vi "日志信息出发送队列 (子VI).vi"(11 "queue out":refnum<queue>) -> (0 "错误输出":errorcluster)   [LabVIEW 2016, in "数据传输系统.lvlib"]
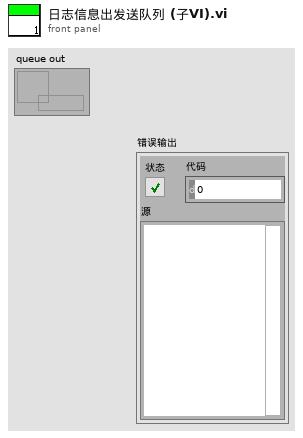
[diagram p1: front panel]
types:
  T1 = enum16{"空白测试", "跨度核查", "标样核查", "加标回收", "平行样", "集成干预"}
  T2 = typedef "数据传输系统.lvlib/应用环境.ctl" = enum16{"STD", "GB212", "婉仪平台"}
  T3 = cluster{"氨氮零点核查索引起始时间":string, "总磷零点核查索引起始时间":string, "总氮零点核查索引起始时间":string, "CODMn零点核查索引起始时间":string, "CODCr零点核查索引起始时间":string, "亚硝酸盐零点核查索引起始时间":string, "硫化物零点核查索引起始时间":string, "ORP零点核查索引起始时间":string, "氟化物零点核查索引起始时间":string, "挥发酚零点核查索引起始时间":string}
  T4 = cluster{"数组[0]":string, "数组[1]":string, "数组[2]":string, "数组[3]":string, "数组[4]":string, "数组[5]":string, "数组[6]":string, "数组[7]":string, "数组[8]":string, "数组[9]":string}
  T5 = cluster{"PH":string[][], "CODCr":string[][], "氨氮":string[][], "CODMn":string[][], "总氮":string[][], "总磷":string[][], "电导率":string[][], "水温":string[][], "DO":string[][], "浊度":string[][], "叶绿素":string[][], "藻密度":string[][], "铜":string[][], "盐度":string[][], "水位":string[][], "流速":string[][], "瞬时流量":string[][], "累积流量":string[][], "亚硝酸盐":string[][], "硫化物":string[][], "ORP":string[][], "铅":string[][], "镉":string[][], "锌":string[][], "镍":string[][], "锰":string[][], "汞":string[][], "气温":string[][], "气压":string[][], "风速":string[][], "风向":string[][], "盐度 2":string[][], "磷酸盐":string[][], "硝氮":string[][], "氟化物":string[][], "挥发酚":string[][], "氯化物":string[][], "蓝绿藻":string[][]}
  T6 = cluster{"氨氮跨度核查索引起始时间":string, "总磷跨度核查索引起始时间":string, "总氮跨度核查索引起始时间":string, "CODMn跨度核查索引起始时间":string, "CODCr跨度核查索引起始时间":string, "亚硝酸盐跨度核查索引起始时间":string, "硫化物跨度核查索引起始时间":string, "ORP跨度核查索引起始时间":string, "氟化物跨度核查索引起始时间":string, "挥发酚跨度核查索引起始时间":string}
  T7 = cluster{"氨氮标样核查索引起始时间":string, "总磷标样核查索引起始时间":string, "总氮标样核查索引起始时间":string, "CODMn标样核查索引起始时间":string, "CODCr标样核查索引起始时间":string, "DO标样核查索引起始时间":string, "PH标样核查索引起始时间":string, "比电导率标样核查索引起始时间":string, "水温标样核查索引起始时间":string, "浊度标样核查索引起始时间":string, "叶绿素a标样核查索引起始时间":string, "藻密度标样核查索引起始时间":string, "亚硝酸盐标样核查索引起始时间":string, "硫化物标样核查索引起始时间":string, "ORP标样核查索引起始时间":string, "氟化物标样核查索引起始时间":string, "挥发酚标样核查索引起始时间":string, "氯化物标样核查索引起始时间":string}
  T8 = cluster{"数组[0]":string, "数组[1]":string, "数组[2]":string, "数组[3]":string, "数组[4]":string, "数组[5]":string, "数组[6]":string, "数组[7]":string, "数组[8]":string, "数组[9]":string, "数组[10]":string, "数组[11]":string, "数组[12]":string, "数组[13]":string, "数组[14]":string, "数组[15]":string, "数组[16]":string, "数组[17]":string}
  T9 = cluster{"氨氮加标回收索引起始时间":string, "总磷加标回收索引起始时间":string, "总氮加标回收索引起始时间":string, "CODMn加标回收索引起始时间":string, "CODCr加标回收索引起始时间":string, "氟化物加标回收索引起始时间":string, "挥发酚加标回收索引起始时间":string}
  T10 = cluster{"[0]":string, "[1]":string, "[2]":string, "[3]":string, "[4]":string, "[5]":string, "[6]":string}
  T11 = cluster{"氨氮平行样索引起始时间":string, "总磷平行样索引起始时间":string, "总氮平行样索引起始时间":string, "CODMn平行样索引起始时间":string, "CODCr平行样索引起始时间":string, "氟化物平行样索引起始时间":string, "挥发酚平行样索引起始时间":string}
  T12 = cluster{"氨氮集成干预索引起始时间":string, "总磷集成干预索引起始时间":string, "总氮集成干预索引起始时间":string, "CODMn集成干预索引起始时间":string, "CODCr集成干预索引起始时间":string, "DO集成干预索引起始时间":string, "PH集成干预索引起始时间":string, "比电导率集成干预索引起始时间":string, "水温集成干预索引起始时间":string, "浊度集成干预索引起始时间":string, "叶绿素a集成干预索引起始时间":string, "藻密度集成干预索引起始时间":string, "亚硝酸盐集成干预索引起始时间":string, "硫化物集成干预索引起始时间":string, "ORP集成干预索引起始时间":string, "氟化物集成干预索引起始时间":string, "挥发酚集成干预索引起始时间":string, "氯化物集成干预索引起始时间":string}
  T13 = cluster{"[0]":string, "[1]":string, "[2]":string, "[3]":string, "[4]":string, "[5]":string, "[6]":string, "[7]":string, "[8]":string, "[9]":string, "[10]":string, "[11]":string, "[12]":string, "[13]":string, "[14]":string, "[15]":string, "[16]":string, "[17]":string}
  T14 = cluster{"氨氮仪器日志索引起始时间":string, "总磷仪器日志索引起始时间":string, "总氮仪器日志索引起始时间":string, "CODMn仪器日志索引起始时间":string, "CODCr仪器日志索引起始时间":string, "系统仪器日志索引起始时间":string, "氟化物仪器日志索引起始时间":string, "挥发酚仪器日志索引起始时间":string}
  T15 = cluster{"[0]":string, "[1]":string, "[2]":string, "[3]":string, "[4]":string, "[5]":string, "[6]":string, "[7]":string}
  T16 = cluster{"氨氮报警信息索引起始时间":string, "总磷报警信息索引起始时间":string, "总氮报警信息索引起始时间":string, "CODMn报警信息索引起始时间":string, "CODCr报警信息索引起始时间":string, "DO报警信息索引起始时间":string, "PH报警信息索引起始时间":string, "比电导率报警信息索引起始时间":string, "水温报警信息索引起始时间":string, "浊度报警信息索引起始时间":string, "叶绿素报警信息索引起始时间":string, "系统报警信息索引起始时间":string, "氟化物报警信息索引起始时间":string, "挥发酚报警信息索引起始时间":string}
  T17 = cluster{"[0]":string, "[1]":string, "[2]":string, "[3]":string, "[4]":string, "[5]":string, "[6]":string, "[7]":string, "[8]":string, "[9]":string, "[10]":string, "[11]":string, "[12]":string, "[13]":string}
  T18 = cluster{"氨氮仪器参数索引起始时间":string, "总磷仪器参数索引起始时间":string, "总氮仪器参数索引起始时间":string, "CODMn仪器参数索引起始时间":string, "CODCr仪器参数索引起始时间":string, "DO仪器参数索引起始时间":string, "PH仪器参数索引起始时间":string, "比电导率仪器参数索引起始时间":string, "水温仪器参数索引起始时间":string, "浊度仪器参数索引起始时间":string, "叶绿素a仪器参数索引起始时间":string, "藻密度仪器参数索引起始时间":string, "ORP仪器参数索引起始时间":string, "氟化物仪器参数索引起始时间":string, "挥发酚仪器参数索引起始时间":string}
  T19 = cluster{"[0]":string, "[1]":string, "[2]":string, "[3]":string, "[4]":string, "[5]":string, "[6]":string, "[7]":string, "[8]":string, "[9]":string, "[10]":string, "[11]":string, "[12]":string, "[13]":string, "[14]":string}
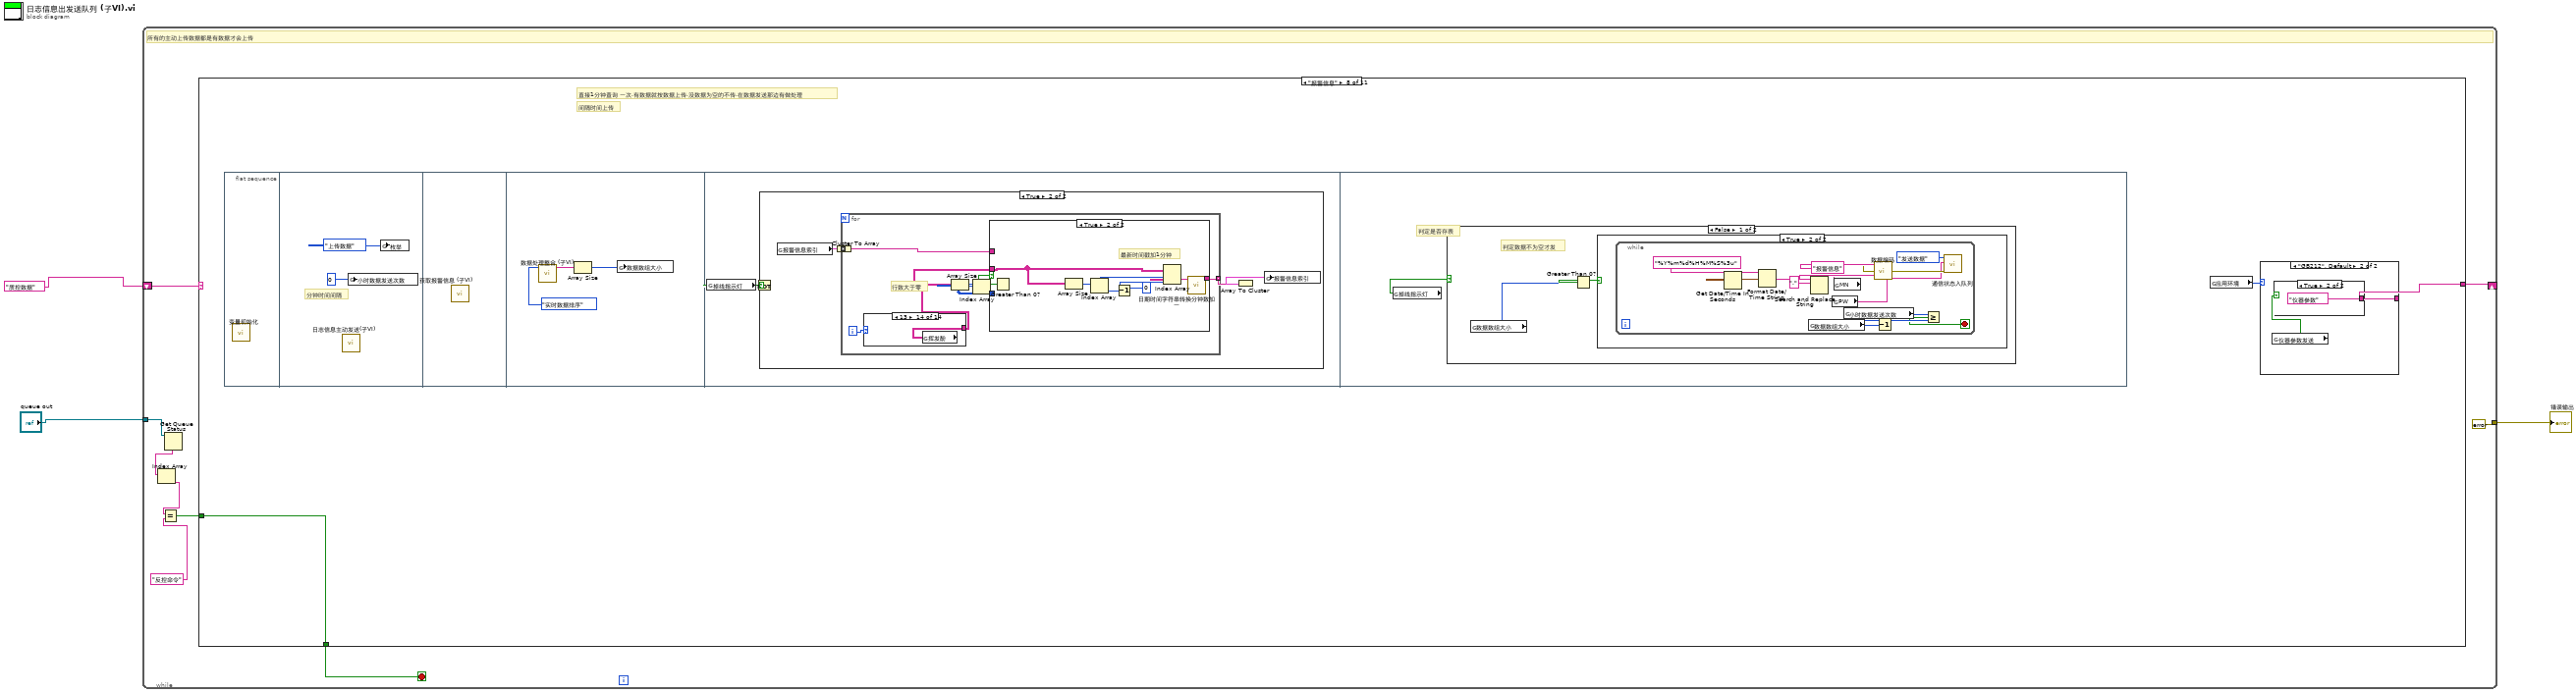
[diagram p0: block diagram]
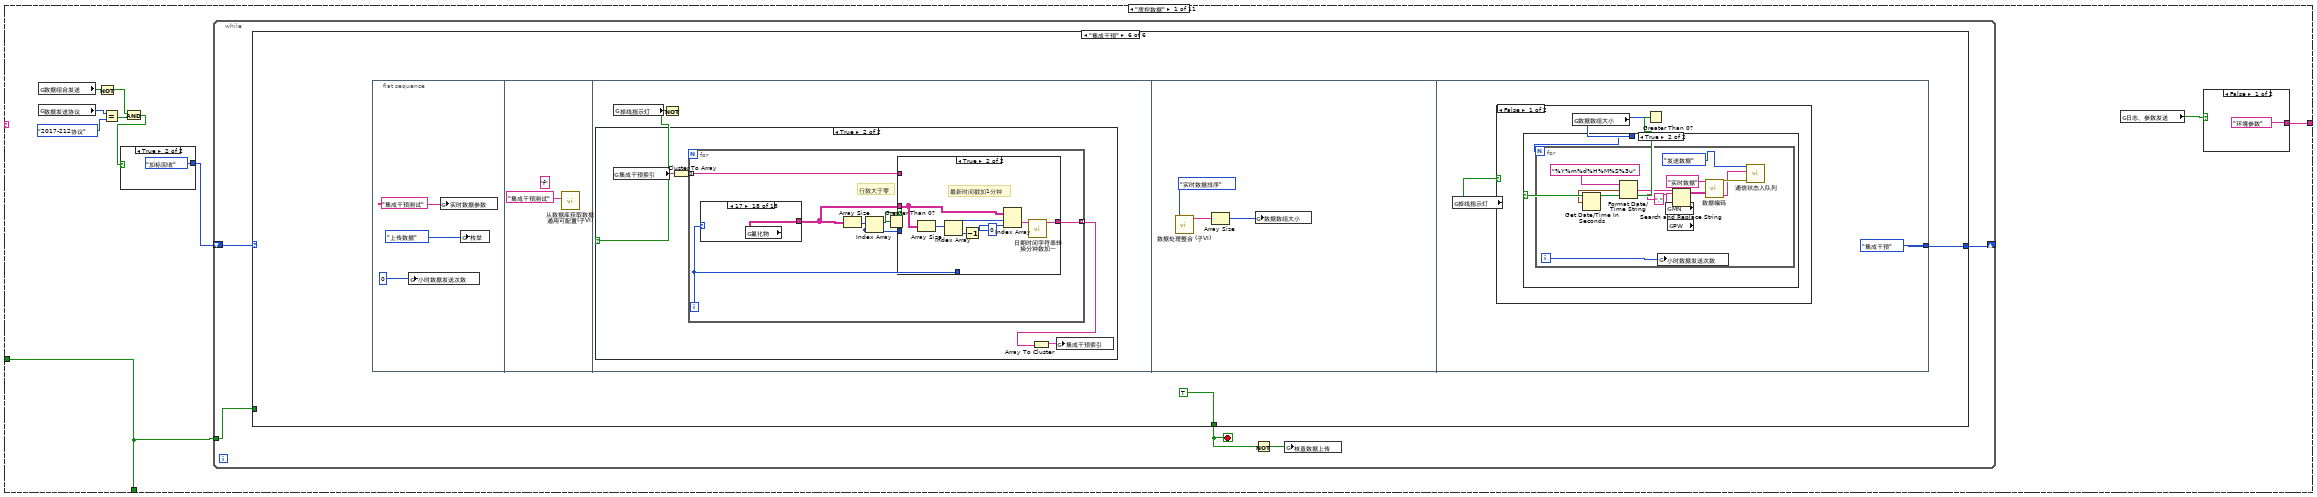
[diagram p2: hidden frame]
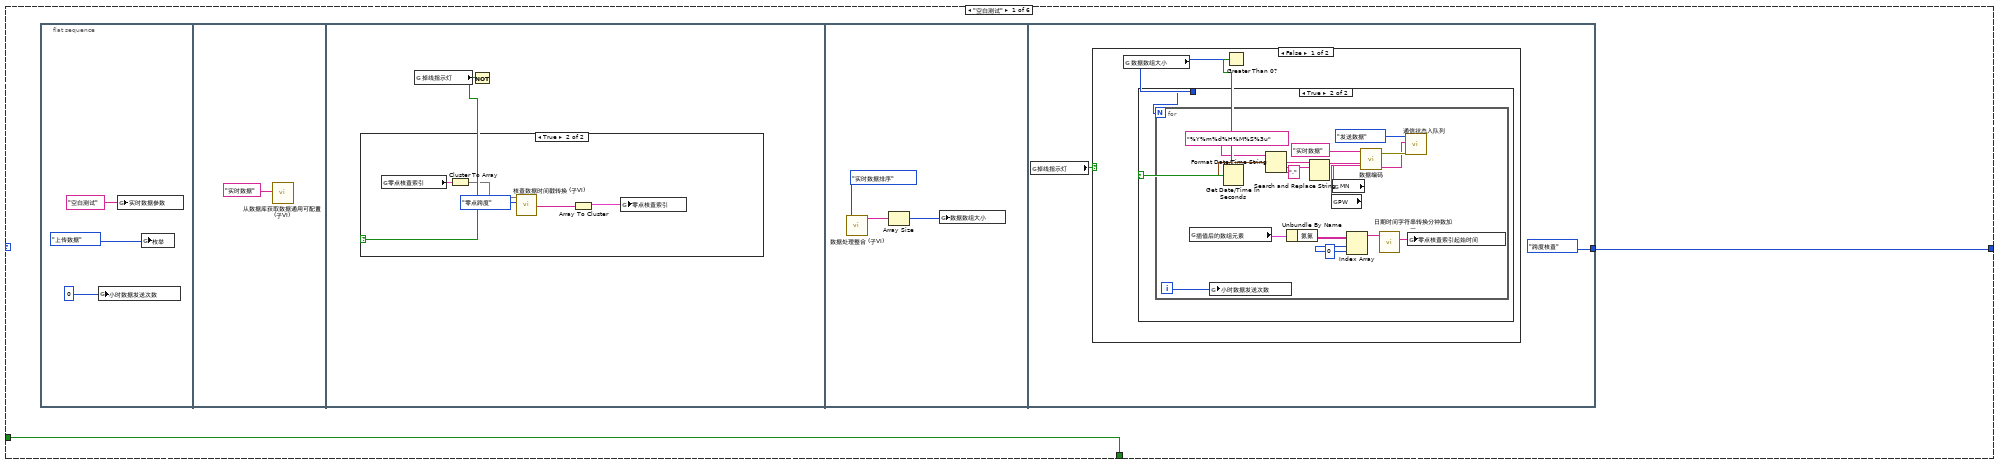
[diagram p3: hidden frame]
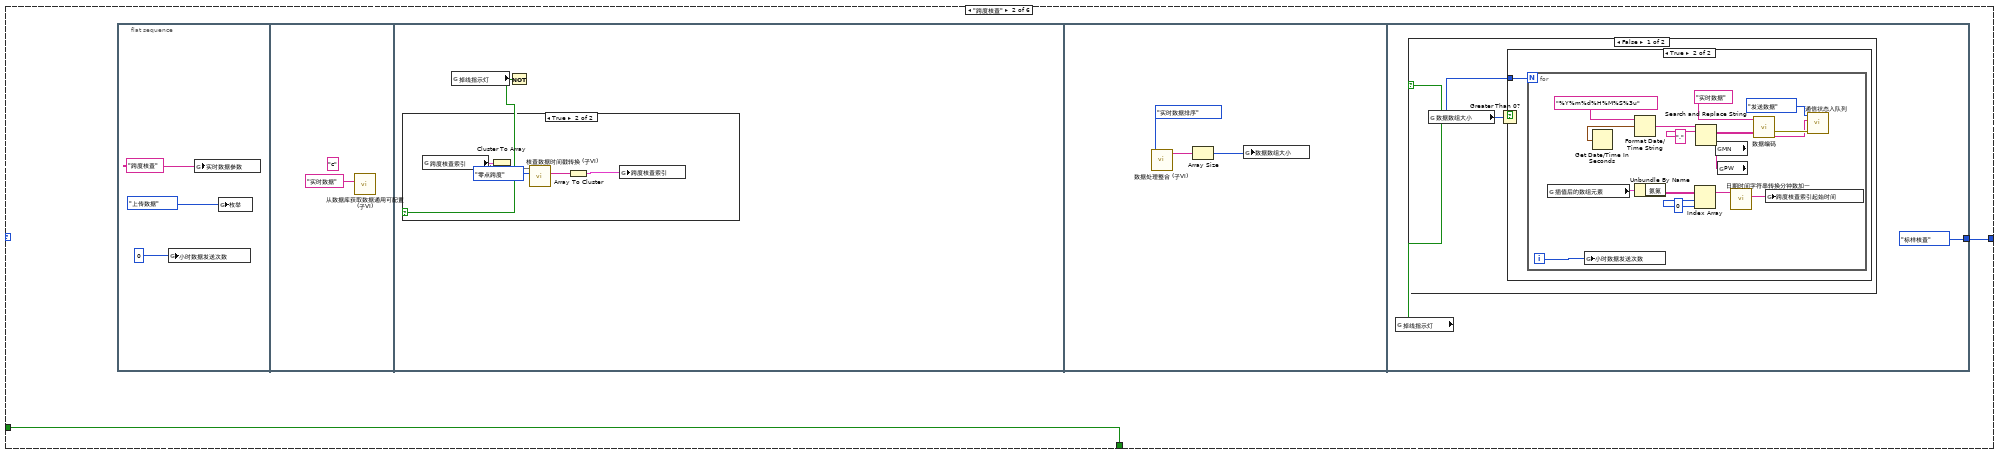
[diagram p7: hidden frame]
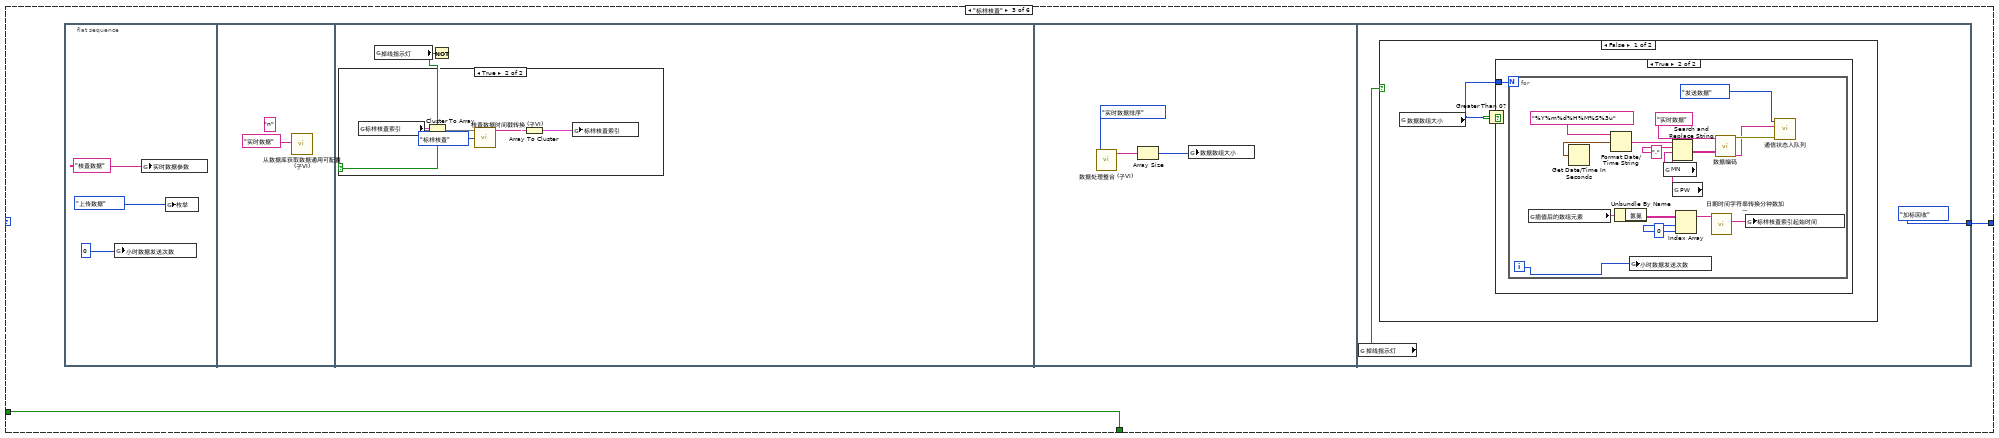
[diagram p11: hidden frame]
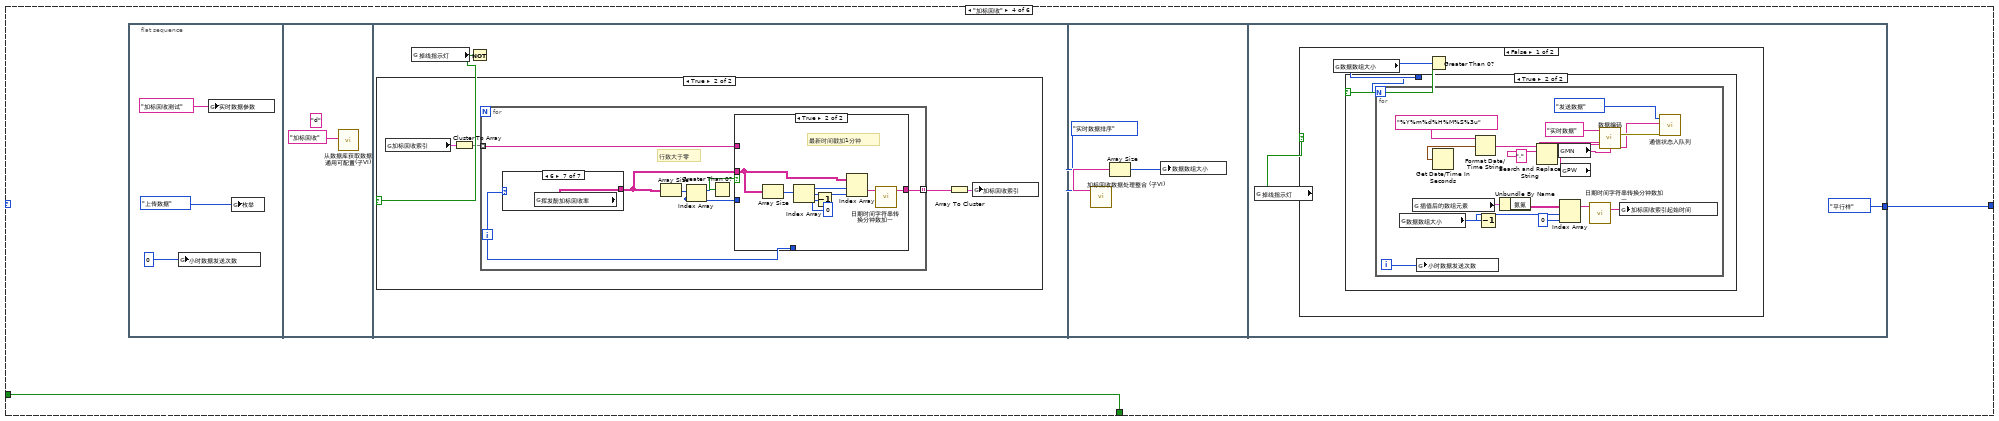
[diagram p15: hidden frame]
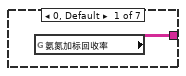
[diagram p17: hidden frame]
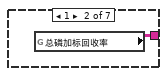
[diagram p18: hidden frame]
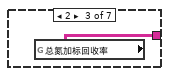
[diagram p19: hidden frame]
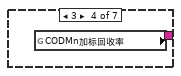
[diagram p20: hidden frame]
diagram:
  n1 = while "While循环" {
    shift-right: [w11] -> _
    shift-left: "质控数据" ("组合框") -> [w12]
    tunnel: [errorcluster {"status"=FALSE, "code"=0, "source"=""} ("错误输出")] -> w3
    tunnel: "queue out" -> [w8]
    stop <- w9 stop-if-true
    # "所有的主动上传数据都是有数据才会上传"
    n2 = Get Queue Status(queue=w8) -> (elements=w7:string[])  [unwired: 2 in, 7 out]
    n3 = Index Array(array=w7) -> (element=w6:string)  [unwired: 1 in]
    n4 = Equal?(x=w6, y="反控命令" ("元素")) -> (x = y?=w4:bool)
    n5 = case shown="\"报警信息\"" w12 {
      tunnel: [w22 w327 "系统状态" ("组合框") w430 "测量周期" ("组合框") "超标留样" ("组合框") "报警信息" ("组合框") w575 w642 "环境参数" ("组合框") "环境参数" ("组合框")] -> w11
      tunnel: [w13 w326 w384 w428 w454 w488 w553 w574 w641 w688 TRUE] -> w9
      tunnel: w4 -> [w13 w326 w384 w428 w454 w488 w553 w574 w641 w688 _]
      frame "质控数据" {
        n6 = global read "断电保存全局.vi" "数据组合发送"() -> (w17:bool)
        n7 = global read "断电保存全局.vi" "数据发送协议"() -> (w20:enum16{"2005-212协议", "2017-212协议"})
        n8 = Not(x=w17) -> (.not. x?=w16:bool)
        n9 = Equal?(x=w20, y=enum16{"2005-212协议", "2017-212协议"}."2017-212协议" ("数据发送协议")) -> (x = y?=w18:bool)
        n10 = And(x=w16, y=w18) -> (x .and. y?=w15:bool)
        n11 = case shown="True" w15 {
          tunnel: [T1."空白测试" T1."加标回收"] -> w14
          frame False {
          }
          frame True {
          }
        }
        n12 = while {
          shift-right: [w26] -> _
          shift-left: w14 -> [w27]
          tunnel: w13 -> [w23]
          stop <- w24 stop-if-true
          n13 = case shown="\"集成干预\"" w27 {
            tunnel: [w28 w66 w104 w142 w203 TRUE] -> w24
            tunnel: [w29 w67 w105 w143 w204 w257] -> w26
            tunnel: w23 -> [w28 w66 w104 w142 w203 _]
            frame "空白测试" {
              n14 = flat-sequence {
                tunnel: [T1."跨度核查"] -> w29
                frame #0 {
                  n15 = global write "全局 小时数据发送次数.vi" "小时数据发送次数"(0 ("小时数据发送次数")) -> ()
                  n16 = global write "全局 实时数据参数.vi" "实时数据参数"("空白测试") -> ()
                  n17 = global write "全局1.vi" "枚举"(enum16{"返回请求应答", "上传数据", "返回执行结果"}."上传数据" ("枚举")) -> ()
                }
                frame #1 {
                  n18 = call "从数据库获取数据通用可配置(子VI).vi"("table输入"="实时数据" ("新元素/子数组")) -> ()  [unwired: 9 in, 2 out]
                }
                frame #2 {
                  n19 = global read "全局 数据发送重叠.vi" "掉线指示灯"() -> (w35:bool)
                  n20 = Not(x=w35) -> (.not. x?=w34:bool)
                  n21 = case shown="True" w34 {
                    frame False {
                    }
                    frame True {
                      n22 = global read "全局 时间2.vi" "零点核查索引"() -> (w40:T3)
                      n23 = Cluster To Array(cluster=w40) -> (array=w38:string[])
                      n24 = call "核查数据时间戳转换 (子VI).vi"("枚举"=enum16{"零点跨度", "标样核查"}."零点跨度", "核查索引"=w38) -> ("数组"=w37:string[])  [unwired: 9 in]
                      n25 = Array To Cluster(array=w37) -> (cluster=w39:T4)
                      n26 = global write "全局 时间2.vi" "零点核查索引"(w39) -> ()
                    }
                  }
                }
                frame #3 {
                  n27 = call "数据处理整合 (子VI).vi"("枚举"=enum16{"实时数据排序", "小时数据排序"}."实时数据排序") -> ("已排序的数组"=w43:string[])  [unwired: 10 in]
                  n28 = Array Size(array=w43) -> (size(s)=w42:i32)
                  n29 = global write "全局 数据数组大小.vi" "数据数组大小"(w42) -> ()
                }
                frame #4 {
                  n30 = global read "全局 数据发送重叠.vi" "掉线指示灯"() -> (w45:bool)
                  n31 = case shown="False" w45 {
                    frame False {
                      n32 = global read "全局 数据数组大小.vi" "数据数组大小"() -> (w46:i32)
                      n33 = Greater Than 0?(x=w46) -> (x > 0?=w47:bool)
                      n34 = case shown="True" w47 {
                        tunnel: w46 -> [_ w48]
                        frame False {
                        }
                        frame True {
                          n35 = for {
                            N: w48 -> [_]
                            i -> [w51]
                            w60 = 0 ("禁用的索引 (列)")
                            n36 = global read "插值后的新数组.vi" "插值后的数组元素"() -> (w64:T5)
                            n37 = global write "全局 小时数据发送次数.vi" "小时数据发送次数"(w51) -> ()
                            n38 = Get Date/Time In Seconds() -> (seconds since 1Jan1904=w55:timestamp)
                            n39 = Format Date/Time String(time format string (%c)="%Y%m%d%H%M%S%3u" ("时间格式字符串(%c)"), seconds (now)=w55) -> (date/time string=w54:string)  [unwired: 1 in]
                            n40 = Unbundle By Name(w64) -> ("氨氮"=w63:string[][])
                            n41 = Search and Replace String(input string=w54, search string="." ("搜索字符串")) -> (result string=w52:string)  [unwired: 6 in, 3 out]
                            n42 = global read "断电保存全局.vi" "PW"() -> (w58:string)
                            n43 = global read "断电保存全局.vi" "MN"() -> (w59:string)
                            n44 = Index Array(array=w63, index (row)=w60, index (col)=w60) -> (element=w62:string)
                            n45 = call "数据编码.vi"("table输入"="实时数据" ("新元素/子数组"), "QN"=w52, "MN"=w59, "PW"=w58) -> ("错误常量"=w57:errorcluster, "通讯包字符串"=w49:string)  [unwired: 10 in]
                            n46 = call "日期时间字符串转换分钟数加一.vi"("data[0]"=w62) -> ("日期/时间字符串"=w61:string)  [unwired: 10 in]
                            n47 = call "通信状态入队列.vi"("错误输入（无错误）"=w57, "发送报文"=w49, "枚举"=enum16{"打开连接", "发送数据", "读取数据", "数据处理", "关闭连接"}."发送数据") -> ()  [unwired: 8 in, 1 out]
                            n48 = global write "全局 时间2.vi" "零点核查索引起始时间"(w61) -> ()
                          }
                        }
                      }
                    }
                    frame True {
                    }
                  }
                }
              }
            }
            frame "跨度核查" {
              n49 = flat-sequence {
                tunnel: [T1."标样核查"] -> w67
                frame #0 {
                  n50 = global write "全局 小时数据发送次数.vi" "小时数据发送次数"(0 ("小时数据发送次数")) -> ()
                  n51 = global write "全局 实时数据参数.vi" "实时数据参数"("跨度核查") -> ()
                  n52 = global write "全局1.vi" "枚举"(enum16{"返回请求应答", "上传数据", "返回执行结果"}."上传数据" ("枚举")) -> ()
                }
                frame #1 {
                  (unwired) "c" ("列队名（唯一）")
                  n53 = call "从数据库获取数据通用可配置(子VI).vi"("table输入"="实时数据" ("新元素/子数组")) -> ()  [unwired: 9 in, 2 out]
                }
                frame #2 {
                  n54 = global read "全局 数据发送重叠.vi" "掉线指示灯"() -> (w73:bool)
                  n55 = Not(x=w73) -> (.not. x?=w72:bool)
                  n56 = case shown="True" w72 {
                    frame False {
                    }
                    frame True {
                      n57 = global read "全局 时间2.vi" "跨度核查索引"() -> (w78:T6)
                      n58 = Cluster To Array(cluster=w78) -> (array=w76:string[])
                      n59 = call "核查数据时间戳转换 (子VI).vi"("枚举"=enum16{"零点跨度", "标样核查"}."零点跨度", "核查索引"=w76) -> ("数组"=w75:string[])  [unwired: 9 in]
                      n60 = Array To Cluster(array=w75) -> (cluster=w77:T4)
                      n61 = global write "全局 时间2.vi" "跨度核查索引"(w77) -> ()
                    }
                  }
                }
                frame #3 {
                  n62 = call "数据处理整合 (子VI).vi"("枚举"=enum16{"实时数据排序", "小时数据排序"}."实时数据排序") -> ("已排序的数组"=w81:string[])  [unwired: 10 in]
                  n63 = Array Size(array=w81) -> (size(s)=w80:i32)
                  n64 = global write "全局 数据数组大小.vi" "数据数组大小"(w80) -> ()
                }
                frame #4 {
                  n65 = global read "全局 数据发送重叠.vi" "掉线指示灯"() -> (w83:bool)
                  n66 = case shown="False" w83 {
                    frame False {
                      n67 = global read "全局 数据数组大小.vi" "数据数组大小"() -> (w84:i32)
                      n68 = Greater Than 0?(x=w84) -> (x > 0?=w85:bool)
                      n69 = case shown="True" w85 {
                        tunnel: w84 -> [_ w86]
                        frame False {
                        }
                        frame True {
                          n70 = for {
                            N: w86 -> [_]
                            i -> [w89]
                            w98 = 0 ("禁用的索引 (列)")
                            n71 = global read "插值后的新数组.vi" "插值后的数组元素"() -> (w102:T5)
                            n72 = global write "全局 小时数据发送次数.vi" "小时数据发送次数"(w89) -> ()
                            n73 = Get Date/Time In Seconds() -> (seconds since 1Jan1904=w93:timestamp)
                            n74 = Format Date/Time String(time format string (%c)="%Y%m%d%H%M%S%3u" ("时间格式字符串(%c)"), seconds (now)=w93) -> (date/time string=w92:string)  [unwired: 1 in]
                            n75 = Unbundle By Name(w102) -> ("氨氮"=w101:string[][])
                            n76 = Index Array(array=w101, index (row)=w98, index (col)=w98) -> (element=w100:string)
                            n77 = Search and Replace String(input string=w92, search string="." ("搜索字符串")) -> (result string=w90:string)  [unwired: 6 in, 3 out]
                            n78 = global read "断电保存全局.vi" "MN"() -> (w97:string)
                            n79 = global read "断电保存全局.vi" "PW"() -> (w96:string)
                            n80 = call "日期时间字符串转换分钟数加一.vi"("data[0]"=w100) -> ("日期/时间字符串"=w99:string)  [unwired: 10 in]
                            n81 = call "数据编码.vi"("table输入"="实时数据" ("新元素/子数组"), "QN"=w90, "MN"=w97, "PW"=w96) -> ("错误常量"=w95:errorcluster, "通讯包字符串"=w87:string)  [unwired: 10 in]
                            n82 = global write "全局 时间2.vi" "跨度核查索引起始时间"(w99) -> ()
                            n83 = call "通信状态入队列.vi"("错误输入（无错误）"=w95, "发送报文"=w87, "枚举"=enum16{"打开连接", "发送数据", "读取数据", "数据处理", "关闭连接"}."发送数据") -> ()  [unwired: 8 in, 1 out]
                          }
                        }
                      }
                    }
                    frame True {
                    }
                  }
                }
              }
            }
            frame "标样核查" {
              n84 = flat-sequence {
                tunnel: [T1."加标回收"] -> w105
                frame #0 {
                  n85 = global write "全局 小时数据发送次数.vi" "小时数据发送次数"(0 ("小时数据发送次数")) -> ()
                  n86 = global write "全局 实时数据参数.vi" "实时数据参数"("核查数据") -> ()
                  n87 = global write "全局1.vi" "枚举"(enum16{"返回请求应答", "上传数据", "返回执行结果"}."上传数据" ("枚举")) -> ()
                }
                frame #1 {
                  (unwired) "n" ("列队名（唯一）")
                  n88 = call "从数据库获取数据通用可配置(子VI).vi"("table输入"="实时数据" ("新元素/子数组")) -> ()  [unwired: 9 in, 2 out]
                }
                frame #2 {
                  n89 = global read "全局 数据发送重叠.vi" "掉线指示灯"() -> (w111:bool)
                  n90 = Not(x=w111) -> (.not. x?=w110:bool)
                  n91 = case shown="True" w110 {
                    frame False {
                    }
                    frame True {
                      n92 = global read "全局 时间2.vi" "标样核查索引"() -> (w116:T7)
                      n93 = Cluster To Array(cluster=w116) -> (array=w114:string[])
                      n94 = call "核查数据时间戳转换 (子VI).vi"("枚举"=enum16{"零点跨度", "标样核查"}."标样核查", "核查索引"=w114) -> ("数组"=w113:string[])  [unwired: 9 in]
                      n95 = Array To Cluster(array=w113) -> (cluster=w115:T8)
                      n96 = global write "全局 时间2.vi" "标样核查索引"(w115) -> ()
                    }
                  }
                }
                frame #3 {
                  n97 = call "数据处理整合 (子VI).vi"("枚举"=enum16{"实时数据排序", "小时数据排序"}."实时数据排序") -> ("已排序的数组"=w119:string[])  [unwired: 10 in]
                  n98 = Array Size(array=w119) -> (size(s)=w118:i32)
                  n99 = global write "全局 数据数组大小.vi" "数据数组大小"(w118) -> ()
                }
                frame #4 {
                  n100 = global read "全局 数据发送重叠.vi" "掉线指示灯"() -> (w121:bool)
                  n101 = case shown="False" w121 {
                    frame False {
                      n102 = global read "全局 数据数组大小.vi" "数据数组大小"() -> (w122:i32)
                      n103 = Greater Than 0?(x=w122) -> (x > 0?=w123:bool)
                      n104 = case shown="True" w123 {
                        tunnel: w122 -> [_ w124]
                        frame False {
                        }
                        frame True {
                          n105 = for {
                            N: w124 -> [_]
                            i -> [w127]
                            w136 = 0 ("禁用的索引 (列)")
                            n106 = global read "插值后的新数组.vi" "插值后的数组元素"() -> (w140:T5)
                            n107 = Get Date/Time In Seconds() -> (seconds since 1Jan1904=w131:timestamp)
                            n108 = Format Date/Time String(time format string (%c)="%Y%m%d%H%M%S%3u" ("时间格式字符串(%c)"), seconds (now)=w131) -> (date/time string=w130:string)  [unwired: 1 in]
                            n109 = Unbundle By Name(w140) -> ("氨氮"=w139:string[][])
                            n110 = global write "全局 小时数据发送次数.vi" "小时数据发送次数"(w127) -> ()
                            n111 = global read "断电保存全局.vi" "MN"() -> (w135:string)
                            n112 = Search and Replace String(input string=w130, search string="." ("搜索字符串")) -> (result string=w128:string)  [unwired: 6 in, 3 out]
                            n113 = global read "断电保存全局.vi" "PW"() -> (w134:string)
                            n114 = Index Array(array=w139, index (row)=w136, index (col)=w136) -> (element=w138:string)
                            n115 = call "日期时间字符串转换分钟数加一.vi"("data[0]"=w138) -> ("日期/时间字符串"=w137:string)  [unwired: 10 in]
                            n116 = call "数据编码.vi"("table输入"="实时数据" ("新元素/子数组"), "QN"=w128, "MN"=w135, "PW"=w134) -> ("错误常量"=w133:errorcluster, "通讯包字符串"=w125:string)  [unwired: 10 in]
                            n117 = global write "全局 时间2.vi" "标样核查索引起始时间"(w137) -> ()
                            n118 = call "通信状态入队列.vi"("错误输入（无错误）"=w133, "发送报文"=w125, "枚举"=enum16{"打开连接", "发送数据", "读取数据", "数据处理", "关闭连接"}."发送数据") -> ()  [unwired: 8 in, 1 out]
                          }
                        }
                      }
                    }
                    frame True {
                    }
                  }
                }
              }
            }
            frame "加标回收" {
              n119 = flat-sequence {
                tunnel: [T1."平行样"] -> w143
                frame #0 {
                  n120 = global write "全局 小时数据发送次数.vi" "小时数据发送次数"(0 ("小时数据发送次数")) -> ()
                  n121 = global write "全局 实时数据参数.vi" "实时数据参数"("加标回收测试") -> ()
                  n122 = global write "全局1.vi" "枚举"(enum16{"返回请求应答", "上传数据", "返回执行结果"}."上传数据" ("枚举")) -> ()
                }
                frame #1 {
                  (unwired) "d" ("列队名（唯一）")
                  n123 = call "从数据库获取数据通用可配置(子VI).vi"("table输入"="加标回收" ("新元素/子数组")) -> ()  [unwired: 9 in, 2 out]
                }
                frame #2 {
                  n124 = global read "全局 数据发送重叠.vi" "掉线指示灯"() -> (w149:bool)
                  n125 = Not(x=w149) -> (.not. x?=w148:bool)
                  n126 = case shown="True" w148 {
                    frame False {
                    }
                    frame True {
                      n127 = global read "全局 时间2.vi" "加标回收索引"() -> (w153:T9)
                      n128 = Cluster To Array(cluster=w153) -> (array=w152:string[])
                      n129 = for {
                        tunnel: [w155] -> w150 mode=indexing
                        tunnel: w152 -> [w154] mode=indexing
                        i -> [w156]
                        # "行数大于零"
                        n130 = case shown="6" w156 {
                          tunnel: [w161 w162 w163 w164 w165 w166 w167] -> w157
                          frame 0, Default {
                            n131 = global read "全局 所有参数.vi" "氨氮加标回收率"() -> (w161:string[][])
                          }
                          frame 1 {
                            n132 = global read "全局 所有参数.vi" "总磷加标回收率"() -> (w162:string[][])
                          }
                          frame 2 {
                            n133 = global read "全局 所有参数.vi" "总氮加标回收率"() -> (w163:string[][])
                          }
                          frame 3 {
                            n134 = global read "全局 所有参数.vi" "CODMn加标回收率"() -> (w164:string[][])
                          }
                          frame 4 {
                            n135 = global read "全局 所有参数.vi" "CODCr加标回收率"() -> (w165:string[][])
                          }
                          frame 5 {
                            n136 = global read "全局 所有参数.vi" "氟化物加标回收率"() -> (w166:string[][])
                          }
                          frame 6 {
                            n137 = global read "全局 所有参数.vi" "挥发酚加标回收率"() -> (w167:string[][])
                          }
                        }
                        n138 = Array Size(array=w157) -> (size(s)=w159:i32[])
                        n139 = Index Array(array=w159) -> (element=w158:i32)  [unwired: 1 in]
                        n140 = Greater Than 0?(x=w158) -> (x > 0?=w160:bool)
                        n141 = case shown="True" w160 {
                          tunnel: w156 -> [_ _]
                          tunnel: w158 -> [_ _]
                          tunnel: w157 -> [_ w172]
                          tunnel: [w168 w169] -> w155
                          tunnel: w154 -> [w168 _]
                          frame False {
                          }
                          frame True {
                            # "最新时间戳加1分钟"
                            n142 = Array Size(array=w172) -> (size(s)=w174:i32[])
                            n143 = Index Array(array=w174) -> (element=w173:i32)  [unwired: 1 in]
                            n144 = Decrement(x=w173) -> (x-1=w171:i32)
                            n145 = Index Array(array=w172, index (row)=w171, index (col)=0 ("禁用的索引 (列)")) -> (element=w175:string)
                            n146 = call "日期时间字符串转换分钟数加一.vi"("data[0]"=w175) -> ("日期/时间字符串"=w169:string)  [unwired: 10 in]
                          }
                        }
                      }
                      n147 = Array To Cluster(array=w150) -> (cluster=w151:T10)
                      n148 = global write "全局 时间2.vi" "加标回收索引"(w151) -> ()
                    }
                  }
                }
                frame #3 {
                  n149 = call "加标回收数据处理整合 (子VI).vi"("枚举"=enum16{"实时数据排序", "小时数据排序"}."实时数据排序") -> ("已排序的数组"=w177:string[])  [unwired: 10 in]
                  n150 = Array Size(array=w177) -> (size(s)=w178:i32)
                  n151 = global write "全局 数据数组大小.vi" "数据数组大小"(w178) -> ()
                }
                frame #4 {
                  n152 = global read "全局 数据发送重叠.vi" "掉线指示灯"() -> (w180:bool)
                  n153 = case shown="False" w180 {
                    frame False {
                      n154 = global read "全局 数据数组大小.vi" "数据数组大小"() -> (w181:i32)
                      n155 = Greater Than 0?(x=w181) -> (x > 0?=w182:bool)
                      n156 = case shown="True" w182 {
                        tunnel: w181 -> [_ w183]
                        frame False {
                        }
                        frame True {
                          n157 = for {
                            N: w183 -> [_]
                            i -> [w186]
                            n158 = global read "全局 数据数组大小.vi" "数据数组大小"() -> (w198:i32)
                            n159 = global read "插值后的新数组.vi" "插值后的数组元素"() -> (w201:T5)
                            n160 = global write "全局 小时数据发送次数.vi" "小时数据发送次数"(w186) -> ()
                            n161 = Get Date/Time In Seconds() -> (seconds since 1Jan1904=w190:timestamp)
                            n162 = Format Date/Time String(time format string (%c)="%Y%m%d%H%M%S%3u" ("时间格式字符串(%c)"), seconds (now)=w190) -> (date/time string=w189:string)  [unwired: 1 in]
                            n163 = Decrement(x=w198) -> (x-1=w197:i32)
                            n164 = Unbundle By Name(w201) -> ("氨氮"=w200:string[][])
                            n165 = Search and Replace String(input string=w189, search string="." ("搜索字符串")) -> (result string=w187:string)  [unwired: 6 in, 3 out]
                            n166 = global read "断电保存全局.vi" "MN"() -> (w194:string)
                            n167 = Index Array(array=w200, index (row)=w197, index (col)=0 ("禁用的索引 (列)")) -> (element=w196:string)
                            n168 = global read "断电保存全局.vi" "PW"() -> (w193:string)
                            n169 = call "日期时间字符串转换分钟数加一.vi"("data[0]"=w196) -> ("日期/时间字符串"=w195:string)  [unwired: 10 in]
                            n170 = call "数据编码.vi"("table输入"="实时数据" ("新元素/子数组"), "QN"=w187, "MN"=w194, "PW"=w193) -> ("错误常量"=w192:errorcluster, "通讯包字符串"=w184:string)  [unwired: 10 in]
                            n171 = global write "全局 时间2.vi" "加标回收索引起始时间"(w195) -> ()
                            n172 = call "通信状态入队列.vi"("错误输入（无错误）"=w192, "发送报文"=w184, "枚举"=enum16{"打开连接", "发送数据", "读取数据", "数据处理", "关闭连接"}."发送数据") -> ()  [unwired: 8 in, 1 out]
                          }
                        }
                      }
                    }
                    frame True {
                    }
                  }
                }
              }
            }
            frame "平行样" {
              n173 = flat-sequence {
                tunnel: [T1."集成干预"] -> w204
                frame #0 {
                  n174 = global write "全局 小时数据发送次数.vi" "小时数据发送次数"(0 ("小时数据发送次数")) -> ()
                  n175 = global write "全局 实时数据参数.vi" "实时数据参数"("平行样测试") -> ()
                  n176 = global write "全局1.vi" "枚举"(enum16{"返回请求应答", "上传数据", "返回执行结果"}."上传数据" ("枚举")) -> ()
                }
                frame #1 {
                  (unwired) "e" ("列队名（唯一）")
                  n177 = call "从数据库获取数据通用可配置(子VI).vi"("table输入"="平行样测试" ("新元素/子数组")) -> ()  [unwired: 9 in, 2 out]
                }
                frame #2 {
                  n178 = global read "全局 数据发送重叠.vi" "掉线指示灯"() -> (w210:bool)
                  n179 = Not(x=w210) -> (.not. x?=w209:bool)
                  n180 = case shown="True" w209 {
                    frame False {
                    }
                    frame True {
                      n181 = global read "全局 时间2.vi" "平行样索引"() -> (w214:T11)
                      n182 = Cluster To Array(cluster=w214) -> (array=w213:string[])
                      n183 = for {
                        tunnel: [w216] -> w211 mode=indexing
                        tunnel: w213 -> [w215] mode=indexing
                        i -> [w217]
                        # "行数大于零"
                        n184 = case shown="6" w217 {
                          tunnel: [w222 w223 w224 w225 w226 w227 w228] -> w218
                          frame 0, Default {
                            n185 = global read "全局 所有参数.vi" "氨氮"() -> (w222:string[][])
                          }
                          frame 1 {
                            n186 = global read "全局 所有参数.vi" "总磷"() -> (w223:string[][])
                          }
                          frame 2 {
                            n187 = global read "全局 所有参数.vi" "总氮"() -> (w224:string[][])
                          }
                          frame 3 {
                            n188 = global read "全局 所有参数.vi" "CODMn"() -> (w225:string[][])
                          }
                          frame 4 {
                            n189 = global read "全局 所有参数.vi" "CODCr"() -> (w226:string[][])
                          }
                          frame 5 {
                            n190 = global read "全局 所有参数.vi" "氟化物"() -> (w227:string[][])
                          }
                          frame 6 {
                            n191 = global read "全局 所有参数.vi" "挥发酚"() -> (w228:string[][])
                          }
                        }
                        n192 = Array Size(array=w218) -> (size(s)=w220:i32[])
                        n193 = Index Array(array=w220) -> (element=w219:i32)  [unwired: 1 in]
                        n194 = Greater Than 0?(x=w219) -> (x > 0?=w221:bool)
                        n195 = case shown="True" w221 {
                          tunnel: w217 -> [_ _]
                          tunnel: w219 -> [_ _]
                          tunnel: w218 -> [_ w233]
                          tunnel: [w229 w230] -> w216
                          tunnel: w215 -> [w229 _]
                          frame False {
                          }
                          frame True {
                            # "最新时间戳加1分钟"
                            n196 = Array Size(array=w233) -> (size(s)=w235:i32[])
                            n197 = Index Array(array=w235) -> (element=w234:i32)  [unwired: 1 in]
                            n198 = Decrement(x=w234) -> (x-1=w232:i32)
                            n199 = Index Array(array=w233, index (row)=w232, index (col)=0 ("禁用的索引 (列)")) -> (element=w236:string)
                            n200 = call "日期时间字符串转换分钟数加一.vi"("data[0]"=w236) -> ("日期/时间字符串"=w230:string)  [unwired: 10 in]
                          }
                        }
                      }
                      n201 = Array To Cluster(array=w211) -> (cluster=w212:T10)
                      n202 = global write "全局 时间2.vi" "平行样索引"(w212) -> ()
                    }
                  }
                }
                frame #3 {
                  n203 = call "数据处理整合 (子VI).vi"("枚举"=enum16{"实时数据排序", "小时数据排序"}."实时数据排序") -> ("已排序的数组"=w239:string[])  [unwired: 10 in]
                  n204 = Array Size(array=w239) -> (size(s)=w238:i32)
                  n205 = global write "全局 数据数组大小.vi" "数据数组大小"(w238) -> ()
                }
                frame #4 {
                  n206 = global read "全局 数据发送重叠.vi" "掉线指示灯"() -> (w240:bool)
                  n207 = case shown="False" w240 {
                    frame False {
                      n208 = global read "全局 数据数组大小.vi" "数据数组大小"() -> (w242:i32)
                      n209 = Greater Than 0?(x=w242) -> (x > 0?=w243:bool)
                      n210 = case shown="True" w243 {
                        tunnel: w242 -> [_ w244]
                        frame False {
                        }
                        frame True {
                          n211 = for {
                            N: w244 -> [_]
                            i -> [w247]
                            n212 = global write "全局 小时数据发送次数.vi" "小时数据发送次数"(w247) -> ()
                            n213 = Get Date/Time In Seconds() -> (seconds since 1Jan1904=w251:timestamp)
                            n214 = Format Date/Time String(time format string (%c)="%Y%m%d%H%M%S%3u" ("时间格式字符串(%c)"), seconds (now)=w251) -> (date/time string=w250:string)  [unwired: 1 in]
                            n215 = Search and Replace String(input string=w250, search string="." ("搜索字符串")) -> (result string=w248:string)  [unwired: 6 in, 3 out]
                            n216 = global read "断电保存全局.vi" "MN"() -> (w255:string)
                            n217 = global read "断电保存全局.vi" "PW"() -> (w254:string)
                            n218 = call "数据编码.vi"("table输入"="实时数据" ("新元素/子数组"), "QN"=w248, "MN"=w255, "PW"=w254) -> ("错误常量"=w253:errorcluster, "通讯包字符串"=w245:string)  [unwired: 10 in]
                            n219 = call "通信状态入队列.vi"("错误输入（无错误）"=w253, "发送报文"=w245, "枚举"=enum16{"打开连接", "发送数据", "读取数据", "数据处理", "关闭连接"}."发送数据") -> ()  [unwired: 8 in, 1 out]
                          }
                        }
                      }
                    }
                    frame True {
                    }
                  }
                }
              }
            }
            frame "集成干预" {
              n220 = flat-sequence {
                tunnel: [T1."集成干预"] -> w257
                frame #0 {
                  n221 = global write "全局 小时数据发送次数.vi" "小时数据发送次数"(0 ("小时数据发送次数")) -> ()
                  n222 = global write "全局 实时数据参数.vi" "实时数据参数"("集成干预测试") -> ()
                  n223 = global write "全局1.vi" "枚举"(enum16{"返回请求应答", "上传数据", "返回执行结果"}."上传数据" ("枚举")) -> ()
                }
                frame #1 {
                  (unwired) "f" ("列队名（唯一）")
                  n224 = call "从数据库获取数据通用可配置(子VI).vi"("table输入"="集成干预测试" ("新元素/子数组")) -> ()  [unwired: 9 in, 2 out]
                }
                frame #2 {
                  n225 = global read "全局 数据发送重叠.vi" "掉线指示灯"() -> (w264:bool)
                  n226 = Not(x=w264) -> (.not. x?=w263:bool)
                  n227 = case shown="True" w263 {
                    frame False {
                    }
                    frame True {
                      n228 = global read "全局 时间2.vi" "集成干预索引"() -> (w268:T12)
                      n229 = Cluster To Array(cluster=w268) -> (array=w267:string[])
                      n230 = for {
                        tunnel: [w270] -> w266 mode=indexing
                        tunnel: w267 -> [w269] mode=indexing
                        i -> [w271]
                        # "行数大于零"
                        n231 = case shown="17" w271 {
                          tunnel: [w276 w277 w278 w279 w280 w281 w282 w283 w284 w285 w286 w287 w288 w289 w290 w291 w292 w293] -> w272
                          frame 0, Default {
                            n232 = global read "全局 所有参数.vi" "氨氮"() -> (w276:string[][])
                          }
                          frame 1 {
                            n233 = global read "全局 所有参数.vi" "总磷"() -> (w277:string[][])
                          }
                          frame 2 {
                            n234 = global read "全局 所有参数.vi" "总氮"() -> (w278:string[][])
                          }
                          frame 3 {
                            n235 = global read "全局 所有参数.vi" "CODMn"() -> (w279:string[][])
                          }
                          frame 4 {
                            n236 = global read "全局 所有参数.vi" "CODCr"() -> (w280:string[][])
                          }
                          frame 5 {
                            n237 = global read "全局 所有参数.vi" "DO"() -> (w281:string[][])
                          }
                          frame 6 {
                            n238 = global read "全局 所有参数.vi" "PH"() -> (w282:string[][])
                          }
                          frame 7 {
                            n239 = global read "全局 所有参数.vi" "电导率"() -> (w283:string[][])
                          }
                          frame 8 {
                            n240 = global read "全局 所有参数.vi" "水温"() -> (w284:string[][])
                          }
                          frame 9 {
                            n241 = global read "全局 所有参数.vi" "浊度"() -> (w285:string[][])
                          }
                          frame 10 {
                            n242 = global read "全局 所有参数.vi" "叶绿素"() -> (w286:string[][])
                          }
                          frame 11 {
                            n243 = global read "全局 所有参数.vi" "藻密度"() -> (w287:string[][])
                          }
                          frame 12 {
                            n244 = global read "全局 所有参数.vi" "亚硝酸盐"() -> (w288:string[][])
                          }
                          frame 13 {
                            n245 = global read "全局 所有参数.vi" "硫化物"() -> (w289:string[][])
                          }
                          frame 14 {
                            n246 = global read "全局 所有参数.vi" "ORP"() -> (w290:string[][])
                          }
                          frame 15 {
                            n247 = global read "全局 所有参数.vi" "氟化物"() -> (w291:string[][])
                          }
                          frame 16 {
                            n248 = global read "全局 所有参数.vi" "挥发酚"() -> (w292:string[][])
                          }
                          frame 17 {
                            n249 = global read "全局 所有参数.vi" "氯化物"() -> (w293:string[][])
                          }
                        }
                        n250 = Array Size(array=w272) -> (size(s)=w274:i32[])
                        n251 = Index Array(array=w274) -> (element=w273:i32)  [unwired: 1 in]
                        n252 = Greater Than 0?(x=w273) -> (x > 0?=w275:bool)
                        n253 = case shown="True" w275 {
                          tunnel: w271 -> [_ _]
                          tunnel: w273 -> [_ _]
                          tunnel: w272 -> [_ w296]
                          tunnel: [w294 w295] -> w270
                          tunnel: w269 -> [w294 _]
                          frame False {
                          }
                          frame True {
                            # "最新时间戳加1分钟"
                            n254 = Array Size(array=w296) -> (size(s)=w300:i32[])
                            n255 = Index Array(array=w300) -> (element=w299:i32)  [unwired: 1 in]
                            n256 = Decrement(x=w299) -> (x-1=w298:i32)
                            n257 = Index Array(array=w296, index (row)=w298, index (col)=0 ("禁用的索引 (列)")) -> (element=w301:string)
                            n258 = call "日期时间字符串转换分钟数加一.vi"("data[0]"=w301) -> ("日期/时间字符串"=w295:string)  [unwired: 10 in]
                          }
                        }
                      }
                      n259 = Array To Cluster(array=w266) -> (cluster=w265:T13)
                      n260 = global write "全局 时间2.vi" "集成干预索引"(w265) -> ()
                    }
                  }
                }
                frame #3 {
                  n261 = call "数据处理整合 (子VI).vi"("枚举"=enum16{"实时数据排序", "小时数据排序"}."实时数据排序") -> ("已排序的数组"=w304:string[])  [unwired: 10 in]
                  n262 = Array Size(array=w304) -> (size(s)=w303:i32)
                  n263 = global write "全局 数据数组大小.vi" "数据数组大小"(w303) -> ()
                }
                frame #4 {
                  n264 = global read "全局 数据发送重叠.vi" "掉线指示灯"() -> (w306:bool)
                  n265 = case shown="False" w306 {
                    frame False {
                      n266 = global read "全局 数据数组大小.vi" "数据数组大小"() -> (w307:i32)
                      n267 = Greater Than 0?(x=w307) -> (x > 0?=w308:bool)
                      n268 = case shown="True" w308 {
                        tunnel: w307 -> [_ w309]
                        frame False {
                        }
                        frame True {
                          n269 = for {
                            N: w309 -> [_]
                            i -> [w312]
                            n270 = Get Date/Time In Seconds() -> (seconds since 1Jan1904=w316:timestamp)
                            n271 = Format Date/Time String(time format string (%c)="%Y%m%d%H%M%S%3u" ("时间格式字符串(%c)"), seconds (now)=w316) -> (date/time string=w315:string)  [unwired: 1 in]
                            n272 = global write "全局 小时数据发送次数.vi" "小时数据发送次数"(w312) -> ()
                            n273 = global read "断电保存全局.vi" "MN"() -> (w319:string)
                            n274 = global read "断电保存全局.vi" "PW"() -> (w318:string)
                            n275 = Search and Replace String(input string=w315, search string="." ("搜索字符串")) -> (result string=w313:string)  [unwired: 6 in, 3 out]
                            n276 = call "数据编码.vi"("table输入"="实时数据" ("新元素/子数组"), "QN"=w313, "MN"=w319, "PW"=w318) -> ("错误常量"=w320:errorcluster, "通讯包字符串"=w310:string)  [unwired: 10 in]
                            n277 = call "通信状态入队列.vi"("错误输入（无错误）"=w320, "发送报文"=w310, "枚举"=enum16{"打开连接", "发送数据", "读取数据", "数据处理", "关闭连接"}."发送数据") -> ()  [unwired: 8 in, 1 out]
                          }
                        }
                      }
                    }
                    frame True {
                    }
                  }
                }
              }
            }
          }
          n278 = Not(x=w24) -> (.not. x?=w25:bool)
          n279 = global write "全局1.vi" "核查数据上传"(w25) -> ()
        }
        n280 = global read "断电保存全局.vi" "日志、参数发送"() -> (w21:bool)
        n281 = case shown="False" w21 {
          tunnel: ["环境参数" ("组合框") "操作日志" ("组合框")] -> w22
          frame False {
          }
          frame True {
          }
        }
      }
      frame "操作日志" {
        # "间隔时间上传"
        # "直接1分钟查询 一次,有数据就按数据上传,没数据就不上传,在数据发送那边有做处理"
        n282 = flat-sequence {
          frame #0 {
            # "时间"
            n283 = global write "全局 小时数据发送次数.vi" "小时数据发送次数"(0 ("小时数据发送次数")) -> ()
            n284 = call "日志信息主动发送(子VI).vi"() -> ()  [unwired: 12 in]
            n285 = global write "全局1.vi" "枚举"(enum16{"返回请求应答", "上传数据", "返回执行结果"}."上传数据" ("枚举")) -> ()
          }
          frame #1 {
            n286 = call "获取操作日志 (子VI).vi"("table输入"="操作日志") -> ()  [unwired: 11 in]
          }
          frame #2 {
            n287 = call "数据处理整合 (子VI).vi"("枚举"=enum16{"实时数据排序", "小时数据排序"}."实时数据排序") -> ("已排序的数组"=w336:string[])  [unwired: 10 in]
            n288 = Array Size(array=w336) -> (size(s)=w335:i32)
            n289 = global write "全局 数据数组大小.vi" "数据数组大小"(w335) -> ()
          }
          frame #3 {
            n290 = global read "全局 数据发送重叠.vi" "掉线指示灯"() -> (w338:bool)
            n291 = Not(x=w338) -> (.not. x?=w337:bool)
            n292 = case shown="True" w337 {
              frame False {
              }
              frame True {
                n293 = global read "全局 时间2.vi" "仪器日志索引"() -> (w342:T14)
                n294 = Cluster To Array(cluster=w342) -> (array=w341:string[])
                n295 = for {
                  tunnel: w341 -> [w343] mode=indexing
                  tunnel: [w344] -> w339 mode=indexing
                  i -> [w346]
                  # "行数大于零"
                  n296 = case shown="7" w346 {
                    tunnel: [w350 w351 w352 w353 w354 w355 w356 w357] -> w345
                    frame 0, Default {
                      n297 = global read "全局 所有参数.vi" "氨氮"() -> (w350:string[][])
                    }
                    frame 1 {
                      n298 = global read "全局 所有参数.vi" "总磷"() -> (w351:string[][])
                    }
                    frame 2 {
                      n299 = global read "全局 所有参数.vi" "总氮"() -> (w352:string[][])
                    }
                    frame 3 {
                      n300 = global read "全局 所有参数.vi" "CODMn"() -> (w353:string[][])
                    }
                    frame 4 {
                      n301 = global read "全局 所有参数.vi" "CODCr"() -> (w354:string[][])
                    }
                    frame 5 {
                      n302 = global read "全局 所有参数.vi" "DO"() -> (w355:string[][])
                    }
                    frame 6 {
                      n303 = global read "全局 所有参数.vi" "氟化物"() -> (w356:string[][])
                    }
                    frame 7 {
                      n304 = global read "全局 所有参数.vi" "挥发酚"() -> (w357:string[][])
                    }
                  }
                  n305 = Array Size(array=w345) -> (size(s)=w348:i32[])
                  n306 = Index Array(array=w348) -> (element=w347:i32)  [unwired: 1 in]
                  n307 = Greater Than 0?(x=w347) -> (x > 0?=w349:bool)
                  n308 = case shown="True" w349 {
                    tunnel: w347 -> [_ _]
                    tunnel: w345 -> [_ w363]
                    tunnel: [w358 w359] -> w344
                    tunnel: w343 -> [w358 _]
                    frame False {
                    }
                    frame True {
                      # "最新时间戳加1分钟"
                      n309 = Array Size(array=w363) -> (size(s)=w365:i32[])
                      n310 = Index Array(array=w365) -> (element=w364:i32)  [unwired: 1 in]
                      n311 = Decrement(x=w364) -> (x-1=w362:i32)
                      n312 = Index Array(array=w363, index (row)=w362, index (col)=0 ("禁用的索引 (列)")) -> (element=w360:string)
                      n313 = call "日期时间字符串转换秒数加一.vi"("data[0]"=w360) -> ("日期/时间字符串"=w359:string)  [unwired: 10 in]
                    }
                  }
                }
                n314 = Array To Cluster(array=w339) -> (cluster=w340:T15)
                n315 = global write "全局 时间2.vi" "仪器日志索引"(w340) -> ()
              }
            }
          }
          frame #4 {
            # "判定是否存表"
            n316 = global read "全局 数据发送重叠.vi" "掉线指示灯"() -> (w366:bool)
            n317 = case shown="False" w366 {
              frame False {
                n318 = global read "全局 数据数组大小.vi" "数据数组大小"() -> (w367:i32)
                n319 = Greater Than 0?(x=w367) -> (x > 0?=w368:bool)
                n320 = case shown="True" w368 {
                  frame False {
                  }
                  frame True {
                    n321 = while {
                      stop <- w369 stop-if-true
                      n322 = Get Date/Time In Seconds() -> (seconds since 1Jan1904=w381:timestamp)
                      n323 = Format Date/Time String(time format string (%c)="%Y%m%d%H%M%S%3u" ("时间格式字符串(%c)"), seconds (now)=w381) -> (date/time string=w380:string)  [unwired: 1 in]
                      n324 = Search and Replace String(input string=w380, search string="." ("搜索字符串")) -> (result string=w378:string)  [unwired: 6 in, 3 out]
                      n325 = global read "断电保存全局.vi" "MN"() -> (w377:string)
                      n326 = global read "断电保存全局.vi" "PW"() -> (w376:string)
                      n327 = call "数据编码.vi"("table输入"="操作日志" ("新元素/子数组"), "QN"=w378, "MN"=w377, "PW"=w376) -> ("错误常量"=w375:errorcluster, "通讯包字符串"=w370:string)  [unwired: 10 in]
                      n328 = global read "全局 小时数据发送次数.vi" "小时数据发送次数"() -> (w372:i32)
                      n329 = global read "全局 数据数组大小.vi" "数据数组大小"() -> (w373:i32)
                      n330 = call "通信状态入队列.vi"("错误输入（无错误）"=w375, "发送报文"=w370, "枚举"=enum16{"打开连接", "发送数据", "读取数据", "数据处理", "关闭连接"}."发送数据") -> ()  [unwired: 8 in, 1 out]
                      n331 = Decrement(x=w373) -> (x-1=w374:i32)
                      n332 = Greater Or Equal?(x=w372, y=w374) -> (x >= y?=w369:bool)
                    }
                  }
                }
              }
              frame True {
              }
            }
          }
        }
        n333 = global read "断电保存全局.vi" "应用环境"() -> (w328:T2)
        n334 = case shown="\"GB212\", Default" w328 {
          tunnel: ["3092日志信息" ("组合框") "系统状态" ("组合框")] -> w327
          frame "STD" {
          }
          frame "GB212", Default {
          }
        }
      }
      frame "3092日志信息" {
        # "间隔时间上传"
        # "直接1分钟查询 一次,有数据就按数据上传,没数据就不上传,在数据发送那边有做处理"
        n335 = flat-sequence {
          tunnel: [w389] -> w385
          tunnel: w385 -> [w393]
          frame #0 {
            n336 = global write "全局 小时数据发送次数.vi" "小时数据发送次数"(0 ("小时数据发送次数")) -> ()
            n337 = global write "全局1.vi" "枚举"(enum16{"返回请求应答", "上传数据", "返回执行结果"}."上传数据" ("枚举")) -> ()
          }
          frame #1 {
            n338 = call "数据表比对.vi"("table输入"="3092日志信息") -> ("待发送数据"=w389:string[][])  [unwired: 7 in, 3 out]
            n339 = global write "全局 所有参数.vi" "CODMn"(w389) -> ()
          }
          frame #2 {
            n340 = Array Size(array=w393) -> (size(s)=w392:i32[])
            n341 = Index Array(array=w392) -> (element=w391:i32)  [unwired: 1 in]
            n342 = global write "全局 数据数组大小.vi" "数据数组大小"(w391) -> ()
          }
          frame #3 {
            n343 = global read "全局 数据发送重叠.vi" "掉线指示灯"() -> (w395:bool)
            n344 = Not(x=w395) -> (.not. x?=w394:bool)
            n345 = case shown="True" w394 {
              frame False {
              }
              frame True {
                # "行数大于零"
                n346 = global read "全局 时间2.vi" "3092日志索引起始时间"() -> (w397:string)
                n347 = global read "全局 所有参数.vi" "CODMn"() -> (w398:string[][])
                n348 = Array Size(array=w398) -> (size(s)=w400:i32[])
                n349 = Index Array(array=w400) -> (element=w399:i32)  [unwired: 1 in]
                n350 = Greater Than 0?(x=w399) -> (x > 0?=w401:bool)
                n351 = case shown="True" w401 {
                  tunnel: w399 -> [_ _]
                  tunnel: w398 -> [_ w407]
                  tunnel: [w402 w403] -> w396
                  tunnel: w397 -> [w402 _]
                  frame False {
                  }
                  frame True {
                    # "最新时间戳加1分钟"
                    n352 = Array Size(array=w407) -> (size(s)=w409:i32[])
                    n353 = Index Array(array=w409) -> (element=w408:i32)  [unwired: 1 in]
                    n354 = Decrement(x=w408) -> (x-1=w406:i32)
                    n355 = Index Array(array=w407, index (row)=w406, index (col)=0 ("禁用的索引 (列)")) -> (element=w404:string)
                    n356 = call "日期时间字符串转换秒数加一.vi"("data[0]"=w404) -> ("日期/时间字符串"=w403:string)  [unwired: 10 in]
                  }
                }
                n357 = global write "全局 时间2.vi" "3092日志索引起始时间"(w396) -> ()
              }
            }
          }
          frame #4 {
            # "判定是否存表"
            n358 = global read "全局 数据发送重叠.vi" "掉线指示灯"() -> (w410:bool)
            n359 = case shown="False" w410 {
              frame False {
                n360 = global read "全局 数据数组大小.vi" "数据数组大小"() -> (w411:i32)
                n361 = Greater Than 0?(x=w411) -> (x > 0?=w412:bool)
                n362 = case shown="True" w412 {
                  frame False {
                  }
                  frame True {
                    n363 = while {
                      stop <- w415 stop-if-true
                      n364 = global read "全局 数据数组大小.vi" "数据数组大小"() -> (w417:i32)
                      n365 = global read "全局 小时数据发送次数.vi" "小时数据发送次数"() -> (w416:i32)
                      n366 = Decrement(x=w417) -> (x-1=w418:i32)
                      n367 = Greater Or Equal?(x=w416, y=w418) -> (x >= y?=w415:bool)
                      n368 = Get Date/Time In Seconds() -> (seconds since 1Jan1904=w425:timestamp)
                      n369 = Format Date/Time String(time format string (%c)="%Y%m%d%H%M%S%3u" ("时间格式字符串(%c)"), seconds (now)=w425) -> (date/time string=w424:string)  [unwired: 1 in]
                      n370 = Search and Replace String(input string=w424, search string="." ("搜索字符串")) -> (result string=w422:string)  [unwired: 6 in, 3 out]
                      n371 = global read "断电保存全局.vi" "MN"() -> (w421:string)
                      n372 = global read "断电保存全局.vi" "PW"() -> (w420:string)
                      n373 = call "数据编码.vi"("table输入"="3092日志信息" ("新元素/子数组"), "QN"=w422, "MN"=w421, "PW"=w420) -> ("错误常量"=w419:errorcluster, "通讯包字符串"=w413:string)  [unwired: 10 in]
                      n374 = call "通信状态入队列.vi"("错误输入（无错误）"=w419, "发送报文"=w413, "枚举"=enum16{"打开连接", "发送数据", "读取数据", "数据处理", "关闭连接"}."发送数据") -> ()  [unwired: 8 in, 1 out]
                    }
                  }
                }
              }
              frame True {
              }
            }
          }
        }
      }
      frame "系统状态" {
        # "直接1分钟查询 一次,有变化就按上传,没变化就不上传"
        n375 = flat-sequence {
          frame #0 {
            # "时间"
            n376 = global write "全局 小时数据发送次数.vi" "小时数据发送次数"(0 ("小时数据发送次数")) -> ()
            n377 = global write "全局 数据数组大小.vi" "数据数组大小"(1 ("数据数组大小")) -> ()
            n378 = global write "全局1.vi" "枚举"(enum16{"返回请求应答", "上传数据", "返回执行结果"}."上传数据" ("枚举")) -> ()
          }
          frame #1 {
            # "判定是否存表"
            n379 = global read "全局 数据发送重叠.vi" "掉线指示灯"() -> (w437:bool)
            n380 = case shown="False" w437 {
              frame False {
                n381 = global read "全局1.vi" "系统状态"() -> (w438:bool)
                n382 = case shown="True" w438 {
                  frame False {
                  }
                  frame True {
                    n383 = for {
                      N: 6 -> [_]
                      n384 = flat-sequence {
                        frame #0 {
                          n385 = Get Date/Time In Seconds() -> (seconds since 1Jan1904=w449:timestamp)
                          n386 = Format Date/Time String(time format string (%c)="%Y%m%d%H%M%S%3u" ("时间格式字符串(%c)"), seconds (now)=w449) -> (date/time string=w448:string)  [unwired: 1 in]
                          n387 = Search and Replace String(input string=w448, search string="." ("搜索字符串")) -> (result string=w446:string)  [unwired: 6 in, 3 out]
                          n388 = global read "断电保存全局.vi" "MN"() -> (w445:string)
                          n389 = global read "断电保存全局.vi" "PW"() -> (w444:string)
                          n390 = call "数据编码.vi"("table输入"="系统状态" ("新元素/子数组"), "QN"=w446, "MN"=w445, "PW"=w444) -> ("错误常量"=w443:errorcluster, "通讯包字符串"=w441:string)  [unwired: 10 in]
                          n391 = call "通信状态入队列.vi"("错误输入（无错误）"=w443, "发送报文"=w441, "枚举"=enum16{"打开连接", "发送数据", "读取数据", "数据处理", "关闭连接"}."发送数据") -> ()  [unwired: 8 in, 1 out]
                        }
                        frame #1 {
                          n392 = global read "全局 小时数据发送次数.vi" "小时数据发送次数"() -> (w453:i32)
                          n393 = Increment(x=w453) -> (x+1=w452:i32)
                          n394 = global write "全局 小时数据发送次数.vi" "小时数据发送次数"(w452) -> ()
                        }
                      }
                    }
                    n395 = global write "全局1.vi" "系统状态"(FALSE ("系统状态")) -> ()
                  }
                }
              }
              frame True {
              }
            }
          }
        }
        n396 = global read "断电保存全局.vi" "应用环境"() -> (w429:T2)
        n397 = case shown="\"GB212\", Default" w429 {
          tunnel: ["运行模式" ("组合框") "超标留样" ("组合框")] -> w430
          frame "STD" {
            n398 = global write "全局 数据发送重叠.vi" "数据接收超时指示灯"(FALSE ("数据接收超时指示灯")) -> ()
          }
          frame "GB212", Default {
          }
        }
      }
      frame "运行模式" {
        # "直接1分钟查询 一次,有变化就按上传,没变化就不上传"
        n399 = flat-sequence {
          frame #0 {
            # "时间"
            n400 = global write "全局 小时数据发送次数.vi" "小时数据发送次数"(0 ("小时数据发送次数")) -> ()
            n401 = global write "全局 数据数组大小.vi" "数据数组大小"(1 ("数据数组大小")) -> ()
            n402 = global write "全局1.vi" "枚举"(enum16{"返回请求应答", "上传数据", "返回执行结果"}."上传数据" ("枚举")) -> ()
          }
          frame #1 {
            # "判定是否存表"
            n403 = global read "全局 数据发送重叠.vi" "掉线指示灯"() -> (w459:bool)
            n404 = case shown="False" w459 {
              frame False {
                n405 = global read "全局1.vi" "运行模式"() -> (w460:bool)
                n406 = case shown="True" w460 {
                  frame False {
                  }
                  frame True {
                    n407 = global read "全局 小时数据发送次数.vi" "小时数据发送次数"() -> (w471:i32)
                    n408 = global write "全局1.vi" "运行模式"(FALSE ("系统状态")) -> ()
                    n409 = Get Date/Time In Seconds() -> (seconds since 1Jan1904=w474:timestamp)
                    n410 = Increment(x=w471) -> (x+1=w470:i32)
                    n411 = Format Date/Time String(time format string (%c)="%Y%m%d%H%M%S%3u" ("时间格式字符串(%c)"), seconds (now)=w474) -> (date/time string=w473:string)  [unwired: 1 in]
                    n412 = global write "全局 小时数据发送次数.vi" "小时数据发送次数"(w470) -> ()
                    n413 = Search and Replace String(input string=w473, search string="." ("搜索字符串")) -> (result string=w465:string)  [unwired: 6 in, 3 out]
                    n414 = global read "断电保存全局.vi" "MN"() -> (w469:string)
                    n415 = global read "断电保存全局.vi" "PW"() -> (w468:string)
                    n416 = call "数据编码.vi"("table输入"="运行模式" ("新元素/子数组"), "QN"=w465, "MN"=w469, "PW"=w468) -> ("错误常量"=w467:errorcluster, "通讯包字符串"=w461:string)  [unwired: 10 in]
                    n417 = call "通信状态入队列.vi"("错误输入（无错误）"=w467, "发送报文"=w461, "枚举"=enum16{"打开连接", "发送数据", "读取数据", "数据处理", "关闭连接"}."发送数据") -> ("错误输出"=w464:errorcluster)  [unwired: 8 in]
                    n418 = global read "断电保存全局.vi" "应用环境"() -> (w463:T2)
                    n419 = case shown="\"STD\"" w463 {
                      tunnel: w465 -> [w480 _]
                      tunnel: w461 -> [w479 _]
                      tunnel: w464 -> [w478 _]
                      frame "STD" {
                        n420 = global read "断电保存全局.vi" "判断数据反馈"() -> (w477:enum16{"非严格判断", "严格判断", "不判断"})
                        n421 = case shown="\"严格判断\"" w477 {
                          tunnel: w479 -> [_ w485]
                          tunnel: w478 -> [_ w484]
                          tunnel: w480 -> [_ w483]
                          frame "不判断", Default {
                          }
                          frame "严格判断" {
                            n422 = global read "断电保存全局.vi" "数据发送通道"() -> (w482:enum16{"TCP", "VISA"})
                            n423 = call "数据补发判定有限循环.vi"("错误输入（无错误）"=w484, "数据输入"=w485, "QN"=w483, "数据发送通道"=w482) -> ("error out"=w481:errorcluster)  [unwired: 7 in]
                            n424 = case shown="No Error" w481 {
                              frame No Error {
                                n425 = global read "全局 数据发送重叠.vi" "数据接收超时指示灯"() -> (w486:bool)
                                n426 = case shown="True" w486 {
                                frame False {
                                }
                                frame True {
                                n427 = global write "全局1.vi" "测量周期"(TRUE ("测量周期")) -> ()
                                }
                                }
                              }
                              frame Error {
                              }
                            }
                          }
                        }
                      }
                      frame "GB212", Default {
                      }
                    }
                  }
                }
              }
              frame True {
              }
            }
          }
        }
      }
      frame "测量周期" {
        # "直接1分钟查询 一次,有变化就按上传,没变化就不上传"
        n428 = flat-sequence {
          frame #0 {
            # "时间"
            n429 = global write "全局 小时数据发送次数.vi" "小时数据发送次数"(0 ("小时数据发送次数")) -> ()
            n430 = global write "全局1.vi" "枚举"(enum16{"返回请求应答", "上传数据", "返回执行结果"}."上传数据" ("枚举")) -> ()
            n431 = global write "全局 数据数组大小.vi" "数据数组大小"(1 ("数据数组大小")) -> ()
          }
          frame #1 {
            # "判定是否存表"
            n432 = global read "全局 数据发送重叠.vi" "掉线指示灯"() -> (w493:bool)
            n433 = case shown="False" w493 {
              frame False {
                n434 = global read "全局1.vi" "测量周期"() -> (w494:bool)
                n435 = case shown="True" w494 {
                  frame False {
                  }
                  frame True {
                    n436 = global read "全局1.vi" "读取各参数测量周期的值"() -> (w502:u16[])
                    n437 = global write "全局1.vi" "测量周期"(FALSE ("系统状态")) -> ()
                    n438 = for {
                      tunnel: w502 -> [w547] mode=indexing
                      shift-right: [w545] -> w506
                      shift-left: u16[] [] ("读取各参数测量周期的值") -> [w548]
                      n439 = Not Equal To 0?(x=w547) -> (x != 0?=w546:bool)
                      n440 = case shown="True" w546 {
                        tunnel: w548 -> [w549 w552]
                        tunnel: w547 -> [_ w551]
                        tunnel: [w549 w550] -> w545
                        frame False {
                        }
                        frame True {
                          n441 = Insert Into Array(array=w552, new element=w551) -> (w550:u16[])  [unwired: 1 in]
                        }
                      }
                    }
                    n442 = global read "断电保存全局.vi" "应用环境"() -> (w500:T2)
                    n443 = Array Max & Min(array=w506) -> (max value=w505:u16, min value=w504:u16)  [unwired: 2 out]
                    n444 = Not Equal?(x=w505, y=w504) -> (x != y?=w507:bool)
                    n445 = Equal?(x=w500, y=应用环境."STD") -> (x = y?=w501:bool)
                    n446 = And(x=w507, y=w501) -> (x .and. y?=w508:bool)
                    n447 = case shown="True" w508 {
                      tunnel: [w524 w536] -> w498
                      tunnel: [w523 w535] -> w497
                      tunnel: [w521 w533] -> w496
                      frame False {
                        n448 = Get Date/Time In Seconds() -> (seconds since 1Jan1904=w530:timestamp)
                        n449 = Format Date/Time String(time format string (%c)="%Y%m%d%H%M%S%3u" ("时间格式字符串(%c)"), seconds (now)=w530) -> (date/time string=w529:string)  [unwired: 1 in]
                        n450 = Search and Replace String(input string=w529, search string="." ("搜索字符串")) -> (result string=w523:string)  [unwired: 6 in, 3 out]
                        n451 = global read "断电保存全局.vi" "MN"() -> (w527:string)
                        n452 = global read "断电保存全局.vi" "PW"() -> (w526:string)
                        n453 = call "数据编码.vi"("table输入"="测量周期" ("新元素/子数组"), "QN"=w523, "MN"=w527, "PW"=w526) -> ("错误常量"=w525:errorcluster, "通讯包字符串"=w521:string)  [unwired: 10 in]
                        n454 = call "通信状态入队列.vi"("错误输入（无错误）"=w525, "发送报文"=w521, "枚举"=enum16{"打开连接", "发送数据", "读取数据", "数据处理", "关闭连接"}."发送数据") -> ("错误输出"=w524:errorcluster)  [unwired: 8 in]
                      }
                      frame True {
                        # "STD&参数测量周期不一样"
                        n455 = Get Date/Time In Seconds() -> (seconds since 1Jan1904=w542:timestamp)
                        n456 = Format Date/Time String(time format string (%c)="%Y%m%d%H%M%S%3u" ("时间格式字符串(%c)"), seconds (now)=w542) -> (date/time string=w541:string)  [unwired: 1 in]
                        n457 = Search and Replace String(input string=w541, search string="." ("搜索字符串")) -> (result string=w535:string)  [unwired: 6 in, 3 out]
                        n458 = global read "断电保存全局.vi" "MN"() -> (w539:string)
                        n459 = global read "断电保存全局.vi" "PW"() -> (w538:string)
                        n460 = call "数据编码.vi"("table输入"="各参数测量周期" ("新元素/子数组"), "QN"=w535, "MN"=w539, "PW"=w538) -> ("错误常量"=w537:errorcluster, "通讯包字符串"=w533:string)  [unwired: 10 in]
                        n461 = call "通信状态入队列.vi"("错误输入（无错误）"=w537, "发送报文"=w533, "枚举"=enum16{"打开连接", "发送数据", "读取数据", "数据处理", "关闭连接"}."发送数据") -> ("错误输出"=w536:errorcluster)  [unwired: 8 in]
                      }
                    }
                    n462 = global read "断电保存全局.vi" "应用环境"() -> (w499:T2)
                    n463 = case shown="\"STD\"" w499 {
                      tunnel: w497 -> [w513 _]
                      tunnel: w496 -> [w512 _]
                      tunnel: w498 -> [w511 _]
                      frame "STD" {
                        n464 = global read "断电保存全局.vi" "判断数据反馈"() -> (w510:enum16{"非严格判断", "严格判断", "不判断"})
                        n465 = case shown="\"严格判断\"" w510 {
                          tunnel: w512 -> [_ w518]
                          tunnel: w511 -> [_ w517]
                          tunnel: w513 -> [_ w516]
                          frame "不判断", Default {
                          }
                          frame "严格判断" {
                            n466 = global read "断电保存全局.vi" "数据发送通道"() -> (w515:enum16{"TCP", "VISA"})
                            n467 = call "数据补发判定有限循环.vi"("错误输入（无错误）"=w517, "数据输入"=w518, "QN"=w516, "数据发送通道"=w515) -> ("error out"=w514:errorcluster)  [unwired: 7 in]
                            n468 = case shown="No Error" w514 {
                              frame No Error {
                                n469 = global read "全局 数据发送重叠.vi" "数据接收超时指示灯"() -> (w519:bool)
                                n470 = case shown="True" w519 {
                                frame False {
                                }
                                frame True {
                                n471 = global write "全局1.vi" "测量周期"(TRUE ("测量周期")) -> ()
                                }
                                }
                              }
                              frame Error {
                              }
                            }
                          }
                        }
                      }
                      frame "GB212", Default {
                      }
                    }
                  }
                }
              }
              frame True {
              }
            }
          }
        }
      }
      frame "超标留样" {
        # "直接1分钟查询 一次,有变化就按上传,没变化就不上传"
        n472 = flat-sequence {
          frame #0 {
            # "时间"
            n473 = global write "全局 小时数据发送次数.vi" "小时数据发送次数"(0 ("小时数据发送次数")) -> ()
            n474 = global write "全局 数据数组大小.vi" "数据数组大小"(1 ("数据数组大小")) -> ()
            n475 = global write "全局1.vi" "枚举"(enum16{"返回请求应答", "上传数据", "返回执行结果"}."上传数据" ("枚举")) -> ()
          }
          frame #1 {
            # "判定是否存表"
            n476 = global read "全局 数据发送重叠.vi" "掉线指示灯"() -> (w558:bool)
            n477 = case shown="False" w558 {
              frame False {
                n478 = global read "全局1.vi" "超标留样"() -> (w559:bool)
                n479 = case shown="True" w559 {
                  frame False {
                  }
                  frame True {
                    n480 = global read "全局 小时数据发送次数.vi" "小时数据发送次数"() -> (w567:i32)
                    n481 = global write "全局1.vi" "超标留样"(FALSE ("系统状态")) -> ()
                    n482 = Get Date/Time In Seconds() -> (seconds since 1Jan1904=w571:timestamp)
                    n483 = Increment(x=w567) -> (x+1=w566:i32)
                    n484 = Format Date/Time String(time format string (%c)="%Y%m%d%H%M%S%3u" ("时间格式字符串(%c)"), seconds (now)=w571) -> (date/time string=w570:string)  [unwired: 1 in]
                    n485 = global write "全局 小时数据发送次数.vi" "小时数据发送次数"(w566) -> ()
                    n486 = Search and Replace String(input string=w570, search string="." ("搜索字符串")) -> (result string=w568:string)  [unwired: 6 in, 3 out]
                    n487 = global read "断电保存全局.vi" "MN"() -> (w564:string)
                    n488 = global read "断电保存全局.vi" "PW"() -> (w563:string)
                    n489 = call "数据编码.vi"("table输入"="超标留样" ("新元素/子数组"), "QN"=w568, "MN"=w564, "PW"=w563) -> ("错误常量"=w565:errorcluster, "通讯包字符串"=w560:string)  [unwired: 10 in]
                    n490 = call "通信状态入队列.vi"("错误输入（无错误）"=w565, "发送报文"=w560, "枚举"=enum16{"打开连接", "发送数据", "读取数据", "数据处理", "关闭连接"}."发送数据") -> ()  [unwired: 8 in, 1 out]
                  }
                }
              }
              frame True {
              }
            }
          }
        }
      }
      frame "报警信息" {
        # "间隔时间上传"
        # "直接1分钟查询 一次,有数据就按数据上传,没数据为空的不传,在数据发送那边有做处理"
        n491 = flat-sequence {
          frame #0 {
            n492 = call "变量初始化.vi"() -> ()  [unwired: 11 in, 1 out]
          }
          frame #1 {
            # "分钟时间间隔"
            n493 = call "日志信息主动发送(子VI).vi"() -> ()  [unwired: 12 in]
            n494 = global write "全局 小时数据发送次数.vi" "小时数据发送次数"(0 ("小时数据发送次数")) -> ()
            n495 = global write "全局1.vi" "枚举"(enum16{"返回请求应答", "上传数据", "返回执行结果"}."上传数据" ("枚举")) -> ()
          }
          frame #2 {
            n496 = call "获取报警信息 (子VI).vi"() -> ()  [unwired: 12 in]
          }
          frame #3 {
            n497 = call "数据处理整合 (子VI).vi"("枚举"=enum16{"实时数据排序", "小时数据排序"}."实时数据排序") -> ("已排序的数组"=w586:string[])  [unwired: 10 in]
            n498 = Array Size(array=w586) -> (size(s)=w585:i32)
            n499 = global write "全局 数据数组大小.vi" "数据数组大小"(w585) -> ()
          }
          frame #4 {
            n500 = global read "全局 数据发送重叠.vi" "掉线指示灯"() -> (w588:bool)
            n501 = Not(x=w588) -> (.not. x?=w587:bool)
            n502 = case shown="True" w587 {
              frame False {
              }
              frame True {
                n503 = global read "全局 时间2.vi" "报警信息索引"() -> (w592:T16)
                n504 = Cluster To Array(cluster=w592) -> (array=w591:string[])
                n505 = for {
                  tunnel: [w594] -> w589 mode=indexing
                  tunnel: w591 -> [w593] mode=indexing
                  i -> [w596]
                  # "行数大于零"
                  n506 = case shown="13" w596 {
                    tunnel: [w600 w601 w602 w603 w604 w605 w606 w607 w608 w609 w610 w611 w612 w613] -> w595
                    frame 0, Default {
                      n507 = global read "全局 所有参数.vi" "氨氮"() -> (w600:string[][])
                    }
                    frame 1 {
                      n508 = global read "全局 所有参数.vi" "总磷"() -> (w601:string[][])
                    }
                    frame 2 {
                      n509 = global read "全局 所有参数.vi" "总氮"() -> (w602:string[][])
                    }
                    frame 3 {
                      n510 = global read "全局 所有参数.vi" "CODMn"() -> (w603:string[][])
                    }
                    frame 4 {
                      n511 = global read "全局 所有参数.vi" "CODCr"() -> (w604:string[][])
                    }
                    frame 5 {
                      n512 = global read "全局 所有参数.vi" "DO"() -> (w605:string[][])
                    }
                    frame 6 {
                      n513 = global read "全局 所有参数.vi" "PH"() -> (w606:string[][])
                    }
                    frame 7 {
                      n514 = global read "全局 所有参数.vi" "电导率"() -> (w607:string[][])
                    }
                    frame 8 {
                      n515 = global read "全局 所有参数.vi" "水温"() -> (w608:string[][])
                    }
                    frame 9 {
                      n516 = global read "全局 所有参数.vi" "浊度"() -> (w609:string[][])
                    }
                    frame 10 {
                      n517 = global read "全局 所有参数.vi" "叶绿素"() -> (w610:string[][])
                    }
                    frame 11 {
                      n518 = global read "全局 所有参数.vi" "藻密度"() -> (w611:string[][])
                    }
                    frame 12 {
                      n519 = global read "全局 所有参数.vi" "氟化物"() -> (w612:string[][])
                    }
                    frame 13 {
                      n520 = global read "全局 所有参数.vi" "挥发酚"() -> (w613:string[][])
                    }
                  }
                  n521 = Array Size(array=w595) -> (size(s)=w598:i32[])
                  n522 = Index Array(array=w598) -> (element=w597:i32)  [unwired: 1 in]
                  n523 = Greater Than 0?(x=w597) -> (x > 0?=w599:bool)
                  n524 = case shown="True" w599 {
                    tunnel: w597 -> [_ _]
                    tunnel: w595 -> [_ w618]
                    tunnel: [w614 w615] -> w594
                    tunnel: w593 -> [w614 _]
                    frame False {
                    }
                    frame True {
                      # "最新时间戳加1分钟"
                      n525 = Array Size(array=w618) -> (size(s)=w620:i32[])
                      n526 = Index Array(array=w620) -> (element=w619:i32)  [unwired: 1 in]
                      n527 = Decrement(x=w619) -> (x-1=w617:i32)
                      n528 = Index Array(array=w618, index (row)=w617, index (col)=0 ("禁用的索引 (列)")) -> (element=w621:string)
                      n529 = call "日期时间字符串转换分钟数加一.vi"("data[0]"=w621) -> ("日期/时间字符串"=w615:string)  [unwired: 10 in]
                    }
                  }
                }
                n530 = Array To Cluster(array=w589) -> (cluster=w590:T17)
                n531 = global write "全局 时间2.vi" "报警信息索引"(w590) -> ()
              }
            }
          }
          frame #5 {
            # "判定是否存表"
            n532 = global read "全局 数据发送重叠.vi" "掉线指示灯"() -> (w622:bool)
            n533 = case shown="False" w622 {
              frame False {
                # "判定数据不为空才发"
                n534 = global read "全局 数据数组大小.vi" "数据数组大小"() -> (w623:i32)
                n535 = Greater Than 0?(x=w623) -> (x > 0?=w624:bool)
                n536 = case shown="True" w624 {
                  frame False {
                    n537 = global write "全局1.vi" "核查数据上传"(FALSE ("数据上传")) -> ()
                  }
                  frame True {
                    n538 = while {
                      stop <- w628 stop-if-true
                      n539 = Get Date/Time In Seconds() -> (seconds since 1Jan1904=w638:timestamp)
                      n540 = Format Date/Time String(time format string (%c)="%Y%m%d%H%M%S%3u" ("时间格式字符串(%c)"), seconds (now)=w638) -> (date/time string=w637:string)  [unwired: 1 in]
                      n541 = global read "全局 数据数组大小.vi" "数据数组大小"() -> (w630:i32)
                      n542 = Search and Replace String(input string=w637, search string="." ("搜索字符串")) -> (result string=w635:string)  [unwired: 6 in, 3 out]
                      n543 = global read "断电保存全局.vi" "PW"() -> (w633:string)
                      n544 = global read "断电保存全局.vi" "MN"() -> (w634:string)
                      n545 = global read "全局 小时数据发送次数.vi" "小时数据发送次数"() -> (w631:i32)
                      n546 = call "数据编码.vi"("table输入"="报警信息" ("新元素/子数组"), "QN"=w635, "MN"=w634, "PW"=w633) -> ("错误常量"=w632:errorcluster, "通讯包字符串"=w626:string)  [unwired: 10 in]
                      n547 = Decrement(x=w630) -> (x-1=w629:i32)
                      n548 = Greater Or Equal?(x=w631, y=w629) -> (x >= y?=w628:bool)
                      n549 = call "通信状态入队列.vi"("错误输入（无错误）"=w632, "发送报文"=w626, "枚举"=enum16{"打开连接", "发送数据", "读取数据", "数据处理", "关闭连接"}."发送数据") -> ()  [unwired: 8 in, 1 out]
                    }
                  }
                }
              }
              frame True {
              }
            }
          }
        }
        n550 = global read "断电保存全局.vi" "应用环境"() -> (w576:T2)
        n551 = case shown="\"GB212\", Default" w576 {
          tunnel: ["3093报警信息" ("组合框") w579] -> w575
          frame "STD" {
          }
          frame "GB212", Default {
            n552 = global read "断电保存全局.vi" "仪器参数发送"() -> (w578:bool)
            n553 = case shown="True" w578 {
              tunnel: ["环境参数" ("组合框") "仪器参数" ("组合框")] -> w579
              frame False {
              }
              frame True {
              }
            }
          }
        }
      }
      frame "3093报警信息" {
        # "间隔时间上传"
        # "直接1分钟查询 一次,有数据就按数据上传,没数据为空的不传,在数据发送那边有做处理"
        n554 = flat-sequence {
          tunnel: [w649] -> w644
          tunnel: w644 -> [w653]
          frame #0 {
            n555 = global write "全局 小时数据发送次数.vi" "小时数据发送次数"(0 ("小时数据发送次数")) -> ()
            n556 = global write "全局1.vi" "枚举"(enum16{"返回请求应答", "上传数据", "返回执行结果"}."上传数据" ("枚举")) -> ()
          }
          frame #1 {
            n557 = call "数据表比对.vi"("table输入"="3093报警信息") -> ("待发送数据"=w649:string[][])  [unwired: 7 in, 3 out]
            n558 = global write "全局 所有参数.vi" "CODMn"(w649) -> ()
          }
          frame #2 {
            n559 = Array Size(array=w653) -> (size(s)=w652:i32[])
            n560 = Index Array(array=w652) -> (element=w651:i32)  [unwired: 1 in]
            n561 = global write "全局 数据数组大小.vi" "数据数组大小"(w651) -> ()
          }
          frame #3 {
            n562 = global read "全局 数据发送重叠.vi" "掉线指示灯"() -> (w655:bool)
            n563 = Not(x=w655) -> (.not. x?=w654:bool)
            n564 = case shown="True" w654 {
              frame False {
              }
              frame True {
                # "行数大于零"
                n565 = global read "全局 时间2.vi" "3093报警索引起始时间"() -> (w657:string)
                n566 = global read "全局 所有参数.vi" "CODMn"() -> (w658:string[][])
                n567 = Array Size(array=w658) -> (size(s)=w660:i32[])
                n568 = Index Array(array=w660) -> (element=w659:i32)  [unwired: 1 in]
                n569 = Greater Than 0?(x=w659) -> (x > 0?=w661:bool)
                n570 = case shown="True" w661 {
                  tunnel: w659 -> [_ _]
                  tunnel: w658 -> [_ w667]
                  tunnel: [w662 w663] -> w656
                  tunnel: w657 -> [w662 _]
                  frame False {
                  }
                  frame True {
                    # "最新时间戳加1分钟"
                    n571 = Array Size(array=w667) -> (size(s)=w669:i32[])
                    n572 = Index Array(array=w669) -> (element=w668:i32)  [unwired: 1 in]
                    n573 = Decrement(x=w668) -> (x-1=w666:i32)
                    n574 = Index Array(array=w667, index (row)=w666, index (col)=0 ("禁用的索引 (列)")) -> (element=w664:string)
                    n575 = call "日期时间字符串转换秒数加一.vi"("data[0]"=w664) -> ("日期/时间字符串"=w663:string)  [unwired: 10 in]
                  }
                }
                n576 = global write "全局 时间2.vi" "3093报警索引起始时间"(w656) -> ()
              }
            }
          }
          frame #4 {
            # "判定是否存表"
            n577 = global read "全局 数据发送重叠.vi" "掉线指示灯"() -> (w670:bool)
            n578 = case shown="False" w670 {
              frame False {
                n579 = global read "全局 数据数组大小.vi" "数据数组大小"() -> (w671:i32)
                n580 = Greater Than 0?(x=w671) -> (x > 0?=w672:bool)
                n581 = case shown="True" w672 {
                  frame False {
                  }
                  frame True {
                    n582 = while {
                      stop <- w675 stop-if-true
                      n583 = global read "全局 数据数组大小.vi" "数据数组大小"() -> (w677:i32)
                      n584 = global read "全局 小时数据发送次数.vi" "小时数据发送次数"() -> (w676:i32)
                      n585 = Decrement(x=w677) -> (x-1=w678:i32)
                      n586 = Greater Or Equal?(x=w676, y=w678) -> (x >= y?=w675:bool)
                      n587 = Get Date/Time In Seconds() -> (seconds since 1Jan1904=w685:timestamp)
                      n588 = Format Date/Time String(time format string (%c)="%Y%m%d%H%M%S%3u" ("时间格式字符串(%c)"), seconds (now)=w685) -> (date/time string=w684:string)  [unwired: 1 in]
                      n589 = Search and Replace String(input string=w684, search string="." ("搜索字符串")) -> (result string=w682:string)  [unwired: 6 in, 3 out]
                      n590 = global read "断电保存全局.vi" "MN"() -> (w681:string)
                      n591 = global read "断电保存全局.vi" "PW"() -> (w680:string)
                      n592 = call "数据编码.vi"("table输入"="3093报警信息" ("新元素/子数组"), "QN"=w682, "MN"=w681, "PW"=w680) -> ("错误常量"=w679:errorcluster, "通讯包字符串"=w673:string)  [unwired: 10 in]
                      n593 = call "通信状态入队列.vi"("错误输入（无错误）"=w679, "发送报文"=w673, "枚举"=enum16{"打开连接", "发送数据", "读取数据", "数据处理", "关闭连接"}."发送数据") -> ()  [unwired: 8 in, 1 out]
                    }
                  }
                }
              }
              frame True {
              }
            }
          }
        }
        n594 = global read "断电保存全局.vi" "仪器参数发送"() -> (w643:bool)
        n595 = case shown="True" w643 {
          tunnel: ["环境参数" ("组合框") "仪器参数" ("组合框")] -> w642
          frame False {
          }
          frame True {
          }
        }
      }
      frame "仪器参数" {
        n596 = flat-sequence {
          frame #0 {
            n597 = global write "全局 小时数据发送次数.vi" "小时数据发送次数"(0 ("小时数据发送次数")) -> ()
            n598 = global write "全局1.vi" "枚举"(enum16{"返回请求应答", "上传数据", "返回执行结果"}."上传数据" ("枚举")) -> ()
          }
          frame #1 {
            n599 = call "获取操作日志 (子VI).vi"("table输入"="仪器参数") -> ()  [unwired: 11 in]
          }
          frame #2 {
            n600 = global read "全局 数据发送重叠.vi" "掉线指示灯"() -> (w694:bool)
            n601 = Not(x=w694) -> (.not. x?=w693:bool)
            n602 = case shown="True" w693 {
              frame False {
              }
              frame True {
                n603 = global read "全局 时间2.vi" "仪器参数索引"() -> (w698:T18)
                n604 = Cluster To Array(cluster=w698) -> (array=w697:string[])
                n605 = for {
                  tunnel: [w702] -> w695 mode=indexing
                  tunnel: w697 -> [w701] mode=indexing
                  i -> [w700]
                  # "行数大于零"
                  n606 = case shown="14" w700 {
                    tunnel: [w706 w707 w708 w709 w710 w711 w712 w713 w714 w715 w716 w717 w718 w719 w720] -> w699
                    frame 0, Default {
                      n607 = global read "全局 所有参数.vi" "氨氮"() -> (w706:string[][])
                    }
                    frame 1 {
                      n608 = global read "全局 所有参数.vi" "总磷"() -> (w707:string[][])
                    }
                    frame 2 {
                      n609 = global read "全局 所有参数.vi" "总氮"() -> (w708:string[][])
                    }
                    frame 3 {
                      n610 = global read "全局 所有参数.vi" "CODMn"() -> (w709:string[][])
                    }
                    frame 4 {
                      n611 = global read "全局 所有参数.vi" "CODCr"() -> (w710:string[][])
                    }
                    frame 5 {
                      n612 = global read "全局 所有参数.vi" "DO"() -> (w711:string[][])
                    }
                    frame 6 {
                      n613 = global read "全局 所有参数.vi" "PH"() -> (w712:string[][])
                    }
                    frame 7 {
                      n614 = global read "全局 所有参数.vi" "电导率"() -> (w713:string[][])
                    }
                    frame 8 {
                      n615 = global read "全局 所有参数.vi" "水温"() -> (w714:string[][])
                    }
                    frame 9 {
                      n616 = global read "全局 所有参数.vi" "浊度"() -> (w715:string[][])
                    }
                    frame 10 {
                      n617 = global read "全局 所有参数.vi" "叶绿素"() -> (w716:string[][])
                    }
                    frame 11 {
                      n618 = global read "全局 所有参数.vi" "藻密度"() -> (w717:string[][])
                    }
                    frame 12 {
                      n619 = global read "全局 所有参数.vi" "ORP"() -> (w718:string[][])
                    }
                    frame 13 {
                      n620 = global read "全局 所有参数.vi" "氟化物"() -> (w719:string[][])
                    }
                    frame 14 {
                      n621 = global read "全局 所有参数.vi" "挥发酚"() -> (w720:string[][])
                    }
                  }
                  n622 = Array Size(array=w699) -> (size(s)=w704:i32[])
                  n623 = Index Array(array=w704) -> (element=w703:i32)  [unwired: 1 in]
                  n624 = Greater Than 0?(x=w703) -> (x > 0?=w705:bool)
                  n625 = case shown="True" w705 {
                    tunnel: w703 -> [_ _]
                    tunnel: w699 -> [_ w726]
                    tunnel: [w721 w723] -> w702
                    tunnel: w701 -> [w721 _]
                    frame False {
                    }
                    frame True {
                      # "最新时间戳加1秒"
                      n626 = Array Size(array=w726) -> (size(s)=w728:i32[])
                      n627 = Index Array(array=w728) -> (element=w727:i32)  [unwired: 1 in]
                      n628 = Decrement(x=w727) -> (x-1=w725:i32)
                      n629 = Index Array(array=w726, index (row)=w725, index (col)=0 ("禁用的索引 (列)")) -> (element=w729:string)
                      n630 = call "日期时间字符串转换分钟数加一.vi"("枚举"=enum16{"分钟数加一", "秒数加一", "小时数加一"}."秒数加一", "data[0]"=w729) -> ("日期/时间字符串"=w723:string)  [unwired: 9 in]
                    }
                  }
                }
                n631 = Array To Cluster(array=w695) -> (cluster=w696:T19)
                n632 = global write "全局 时间2.vi" "仪器参数索引"(w696) -> ()
              }
            }
          }
          frame #3 {
            n633 = global read "全局 数据发送重叠.vi" "掉线指示灯"() -> (w731:bool)
            n634 = Not(x=w731) -> (.not. x?=w730:bool)
            n635 = case shown="True" w730 {
              frame False {
              }
              frame True {
                n636 = call "3020仪器参数发送.vi"() -> ()  [unwired: 12 in]
              }
            }
          }
        }
      }
      frame "环境参数", Default {
        n637 = call "核查数据断电保存 (子VI).vi"() -> ()  [unwired: 12 in]
      }
    }
  }
  "错误输出" <- w3
